vi "RITA_GUI.vi"() -> ()   [LabVIEW 2012]
uses:
  <vilib>/silver_ctls/ArrayMatrixCluster/Real Matrix NI_Silver.ctl
  State.ctl
  Signal Analysis.lvlib
  Report.lvlib
  Logger VIs.lvlib
  Pressure Regulator Controller.lvlib
  MultiClamp 700B Controls.lvlib
  Sciscan Scope Daemon.lvlib
  Autopatcher Daemon.lvlib
  Visual Analyser.lvlib
  Scientifica Manipulator Daemon.lvlib
  Targeting Unit.lvlib
  Signal Acquisition.lvlib
panel:
  in  "Start Coordinates [pix] 2":cluster{"X":dbl, "Y":dbl}
  out "Traced Objects [pix]":T1(array[cluster])
  out "All Objects [pix]":T1(array[cluster])
  in  "Traced Objects":i32
  in  "Start Coordinates [pix]":cluster{"X":dbl, "Y":dbl}
  in  "State":T2=enum."LOAD"
  in  "Autotune Gain":bool
  in  "Target Amplitude [V]":dbl
  in  "Main Tab Control":enum32{"Main", "Report", "Configuration"}(tab)
  in  "Target\nDistance [um]":dbl
  in  "Axial Approach":bool
  in  "Image construction":T3={"Delay"=1.0, "Display-N"=0, "Average"=0, "Frames"=10, "Zoom"=1.0, "Time\nStamp"=timestamp(0 s since 1904-01-01), "Auto Delay"=FALSE} {"Zoom" items=["1X"=1.0, "2X"=2.0, "3X"=3.0, "4X"=4.0, "5X"=5.0, "6X"=6.0, "7X"=7.0, "8X"=8.0]; "Average" items=["No Average", "Group Average", "Moving Average"]; "Delay" min=1.0 max=320.0 step=1.0 scale=1.0..320.0}
  out "Resistance [MOhm]":dbl format="%#_5g"
  out "Current [nA]":dbl format="%#_3g"
  in  "Gain":u16(ring)=1 items=["1"=1, "2"=2, "5"=5, "10"=10, "20"=20, "50"=50, "100"=100, "200"=200, "500"=500, "1000"=1000, "2000"=2000]
  in  "Manipulator":T4={"Indicator 7"={"Approach Indicator"=TRUE}, "Zero"=FALSE, "Step"=FALSE, "Drive to"=FALSE, "Current Position"={"X [um]"=0.0, "Y [um]"=0.0, "Z [um]"=0.0}, "Indicator 15"={"Status"=FALSE}, "Depth [um]"=0.0, "Destination Position"={"X [um]"=0.0, "Y [um]"=0.0, "Z [um]"=0.0}, "Go to"=FALSE, "Axial Approach"=TRUE, "Direction"=enum."Axial"}
  in  "Test Signal Parameters and Offset":T5 {"Frequency\n[hz]" items=["2 hz "=2, "5 hz"=5, "10 hz "=10, "20 hz"=20, "50 hz"=50, "60 hz"=60, "100 hz"=100, "200 hz"=200, "500 hz"=500, "1000 hz"=1000]}
  out "Test Signal":waveform(dbl)(graph)
  out "Resistance":T6(graph)
  out "Current":dbl(graph)
  in  "Pressure Controls":T7 {"Pressure Sp Manual [KPa]" scale=-50.0..100.0}
  in  "Holding Potential":T8 {"Holding Potential [mV]" scale=-100.0..100.0}
  in  "Signal Filter and PSD":T9
  in  "Dialog":cluster{"Indicator":bool}
  in  "High Level Controls":T10={"Record Button"=FALSE, "Exit"=FALSE, "Hunt"=FALSE, "Break In"=FALSE, "Seal"=FALSE, "Drive In"=FALSE, "Load Pipette"=FALSE, "REC"=FALSE, "File Path Control"=path "D:/Rita Logfiles", "Auto Button"=FALSE, "Auto"=FALSE, "Engage Target"=FALSE, "Abort"=FALSE}
  in  "Tip Acquisition":T11={"Focus Tip"=FALSE, "Acquire Tip"=FALSE, "Indicator 7"={"Tip Indicator"=FALSE}, "Tip Coordinates"={"X [um]"=nan, "Y [um]"=nan, "Z [um]"=nan}, "Disengage Tip"=FALSE}
  in  "Target Acquisition":T12={"Indicator 7"={"Target Indicator"=FALSE}, "Focus Target"=FALSE, "Acquire Target"=FALSE, "Target Coordinates"={"X [um]"=nan, "Y [um]"=nan, "Z [um]"=nan}, "Disengage Target"=FALSE}
  in  "Capacitance Compensation":T13
  out "Image":T14(plugin-control)
  in  "Resistance Levels":T15={"R0"=0.0, "R0/R1"=0.0, "R1"=0.0, "R1/R2"=0.0, "R2"=0.0, "R0-R2"=0.0, "R0/R2"=0.0, "Detect [%]"=10.0, "Break in "=100.0} {"Break in" scale=1.0..1000.0; "Detect [%]" scale=1.0..1000.0; "R0/R2" format="%.0f%%"; "R0-R2" scale=-100.0..100.0; "R2" scale=1.0..1000.0; "R1/R2" format="%.0f%%"; "R1" scale=1.0..1000.0; "R0/R1" format="%.0f%%"; "R0" scale=1.0..1000.0}
  in  "Scope Position":T16
  in  "Pipette Crash Indicator":cluster{"Pipette Crash":bool}
  in  "Align Trajectory":bool
  in  "Find Shank":bool
  in  "Find Tip":bool
  in  "Visualization Channels":T17={"Red\nChannel"={-29500.0, 275.0}, "Auto Adjust Red"=TRUE, "Green\nChannel"={-31433.0, -13386.0}, "Auto Adjust Green"=TRUE, "Visualized Color Plane"=8} {"Visualized Color Plane" items=["Red", "Green", "Blue", "Hue", "Saturation", "Luminance", "Value", "Intensity", "RGB"]; "Green\nChannel" scale=-32768.0..32767.0; "Red\nChannel" scale=-32768.0..32767.0}
  in  "Focus Button":bool
  in  "FOV":T18
  in  "Tab Control 2":enum32{"Analysis", "Calibration"}(tab)
  in  "Analisys and Tracking":T19={"Image Analisys"=TRUE, "Analysis\nPlane"=0, "Erosion\nFilter"=4, "Target Update Method"=0, "Objects"=0, "Target Update"=FALSE, "Object Tracking"=FALSE, "Traced\nObject\n[um]"={"X"=nan, "Y"=nan, "Z"=nan}, "Status"=FALSE, "Area"=0.0, "Cntr"=0.0} {"Target Update Method" items=["On Demand", "Continuos"]; "Erosion\nFilter" max=10 step=1 scale=0.0..10.0; "Analysis\nPlane" items=["Red", "Green", "Blue", "Hue", "Saturation", "Luminance", "Value", "Intensity"]}
  in  "Calibration Angles":T20={"Angles"={"Azimut"=-0.02262988105691686, "Elevation"=0.523611383535619}, "Calibrate Azimut"=FALSE, "Calibrate Elevation"=FALSE, "Autocalibration"=FALSE, "Acquire Initial Point"=FALSE, "Acquire Final Point"=FALSE} {"Angles"."Elevation" format="%#_10g"; "Angles"."Azimut" format="%#_10g"}
  in  "FOV Calibration":T21
  in  "Analyzer":bool=TRUE
  in  "Axial distance to cover [um]":dbl
  out "Logo":cluster{"Logo":picture}
  in  "Report Indicator":T22={"Report Plot"=FALSE, "File Path Control"=path "", "Resistance"=[], "Current"=[], "Current 2"=[], "Current 3"=[], "Position"=[], "Slider"=0.0, "Trajectory"=[], "Report Image"=refnum, "Play Button"=FALSE, "Report Visualization Options"={"Red\nChannel"={0.0, 7.070707070707071}, "Auto Adjust Red"=FALSE, "Green\nChannel"={0.0, 7.070707070707071}, "Auto Adjust Green"=FALSE, "Visualized Color Plane"=8, "Vision Overlay"=TRUE}, "Loading Bar"=0.0} {"Loading Bar" min=0.0 max=1.0 step=0.001 scale=0.0..1.0; "Report Visualization Options"."Visualized Color Plane" items=["Red", "Green", "Blue", "Hue", "Saturation", "Luminance", "Value", "Intensity", "RGB"]; "Report Visualization Options"."Green\nChannel" scale=-32768.0..32767.0; "Report Visualization Options"."Red\nChannel" scale=-32768.0..32767.0; "Slider" min=0.0 step=0.05 scale=0.0..600.0}
  in  "Geometrical Transformation Parameters":T24={"Scope Transformation Matrix"=[[1.0, 0.0], [0.0, 1.0]], "Manipulator transformation"=[[-1.0], [-1.0], [-1.0]], "Coorection Factor"={"Kx"=1.0, "Ky"=1.0, "Kz"=1.0}} {"Coorection Factor"."Kz" format="%#_10g"; "Coorection Factor"."Ky" format="%#_10g"; "Coorection Factor"."Kx" format="%#_10g"}
  in  "Calibration Parameters":T25={"Test Signal"={"Break In"={"Amplitude [mV]"=30, "Frequency [hz]"=100}, "Extracellular"={"Amplitude [mV]"=10, "Frequency [hz]"=100}}, "Capacitance Compensation"={"Iterations"=2, "Timeout [ms]"=3000}, "Holding Potential Dynamics"={"Start [mV]"=-70.0, "Target [mV]"=-70.0, "Speed [mV/s]"=2.0}, "Manipulator Dynamics"={"Step length [um]"=2.0, "Interstep Interval [ms]"=1500, "Initial Speed [um/s]"=10.0, "Max Speed [um/s]"=10.0, "Acceleration [um/s^2]"=10.0, "Max Depth [um]"=1200.0, "Max Penetration [um]"=1200.0}, "Suction Parameters"={"Initial Pressure [Kpa]"=-5.0, "Minimum Pressure [KPa]"=-25.0, "Decremental Step [KPa]"=-5.0, "Decremental Threshold [%]"=5.0, "Falloff Threshold [%]"=50.0, "Falloff Lag [ms]"=3000.0, "Monitor Refresh [ms]"=1000.0}, "Pressure SPs [KPa]"={"High"=50.0, "Low"=10.0}, "Seal Parameters"={"Seal Target [MOhm]"=1000.0, "Stability Threhsold [%]"=10.0, "Seal Timeout [s]"=600.0, "Stability Refresh [ms]"=1000.0}, "Break in pulse Dynamics"={"Length [ms]"=250.0, "Voltage [mV]"=1000.0, "Pressure [KPa]"=-25.0}, "Unblockage Parameters"={"Blockage Threshold [%]"=10.0, "Max Attempt"=3}, "Targeter Settings"={"Approaching Calibration"={"Approach Factor [um]"=0.9, "Final Clearance [um]"=2.0}, "Optic Flow Settings"={"Pyramid Levels"=6, "Max Iterations"=8, "Displacement Threshold"=0.0, "Window Size"=45}, "Focus"={"Timeout [ms]"=5000, "Max Attempts"=2, "Method"=enum."Continuous"}}} {"Test Signal"."Extracellular"."Frequency [hz]" items=["2 hz "=2, "5 hz"=5, "10 hz "=10, "20 hz"=20, "50 hz"=50, "60 hz"=60, "100 hz"=100, "200 hz"=200, "500 hz"=500, "1000 hz"=1000]; "Test Signal"."Break In"."Frequency [hz]" items=["2 hz "=2, "5 hz"=5, "10 hz "=10, "20 hz"=20, "50 hz"=50, "60 hz"=60, "100 hz"=100, "200 hz"=200, "500 hz"=500, "1000 hz"=1000]}
  in  "Hardware Configuration":T26={"Pressure Controller Dynamics"={"Positive Branch"={"Kp"=0.05, "Ki"=1.0, "Kd"=1e-06}, "Negative Branch"={"Kp"=1.0, "Ki"=10.0, "Kd"=1e-06}}, "Amplifier"={"Multiclamp Serial Number"="00832548", "Multiclamp Channel"=0}, "Manipulator Port"="COM10", "Objective"=600, "Sciscan core Ref"=path "C:/Users/Southampton/Desktop/LUCA_SciScan_141211/GFG/GFG_core.ref", "Signals Sampling"={"Sample Mode"=10123, "Sampling frequecy [hz]"=20000.0, "Samples Number"=1000}, "Electrode Signals"={"Scale Type"=10348, "Terminal Configuration"=10083, "Scale Name"="", "Range [V]"={"max"=10.0, "min"=-10.0}, "Channel 2 [Potential]"="Dev4/ai1", "Channel 1 [Current]"="Dev4/ai2"}, "Pressure Signal"={"Scale Type"=10065, "Terminal Configuration"=10083, "Scale Name"="Compund Pressure", "Range [V]"={"max"=4.0, "min"=0.0}, "Physical Channel"="Dev4/ai4"}, "IIR Filter Specifications"={"Topology"=enum."Off", "Type"=enum."Lowpass", "Order"=0, "Lower Fc"=0.0, "Upper Fc"=0.0, "PB Ripple"=0.0, "SB Attenuation"=0.0}, "Pressure Controller Port"="COM8", "Scope Dynamics"={"Initial Speed [um/s]"=500.0, "Max Speed [um/s]"=1000.0, "Acceleration [um/s^2]"=25.0, "Max Depth [um]"=5000.0}} {"Pressure Signal"."Terminal Configuration" items=["Default"=-1, "RSE"=10083, "Differential"=10106, "Pseudodifferential"=12529]; "Pressure Signal"."Scale Type" items=["Volts"=10348, "Custom Scale"=10065]; "Electrode Signals"."Terminal Configuration" items=["Default"=-1, "RSE"=10083, "Differential"=10106, "Pseudodifferential"=12529]; "Electrode Signals"."Scale Type" items=["Volts"=10348, "Custom Scale"=10065]; "Signals Sampling"."Sample Mode" items=["Finite Samples"=10178, "Continuous Samples"=10123, "Hardware Timed Single Point"=12522]; "Objective" items=["Nikon 16x / 0.80w"=600]; "Amplifier"."Multiclamp Channel" items=["Channel 1", "Channel 2"]}
  in  "Pipette Search":T27={"Stability Delay [ms]"=1000, "Scan Area"={"Lateral [um]"=1200.0, "Vertical [um]"=1600.0}, "Vertical Sections"=10, "Scanning Direction"={"X"=0, "Y"=1, "Z"=1}, "Fucusing step [um]"=-30.0, "Erosion Value"=3} {"Scanning Direction"."Z" items=["Negative"=-1, "Positive"=1]; "Scanning Direction"."Y" items=["Negative"=-1, "Fixed"=0, "Positive"=1]; "Scanning Direction"."X" items=["Negative"=-1, "Fixed"=0, "Positive"=1]}
  in  "Configuration Files":T28
  out "Error Out":errorcluster
  # "Image"
  # "Test signal and offset"
  # "Capacitance Compensation"
  # "Visualization"
  # "Analysis and Tracking"
  # "Calibration Angles"
  # "Visualization"
  # "Xv"
  # "Yv"
  # "Xscope"
  # "Yscope"
  # "axial direction (exiting -1 entering +1)"
  # "Flip System of Reference (Yes -1 No 1)"
  # "Insertion step Sign"
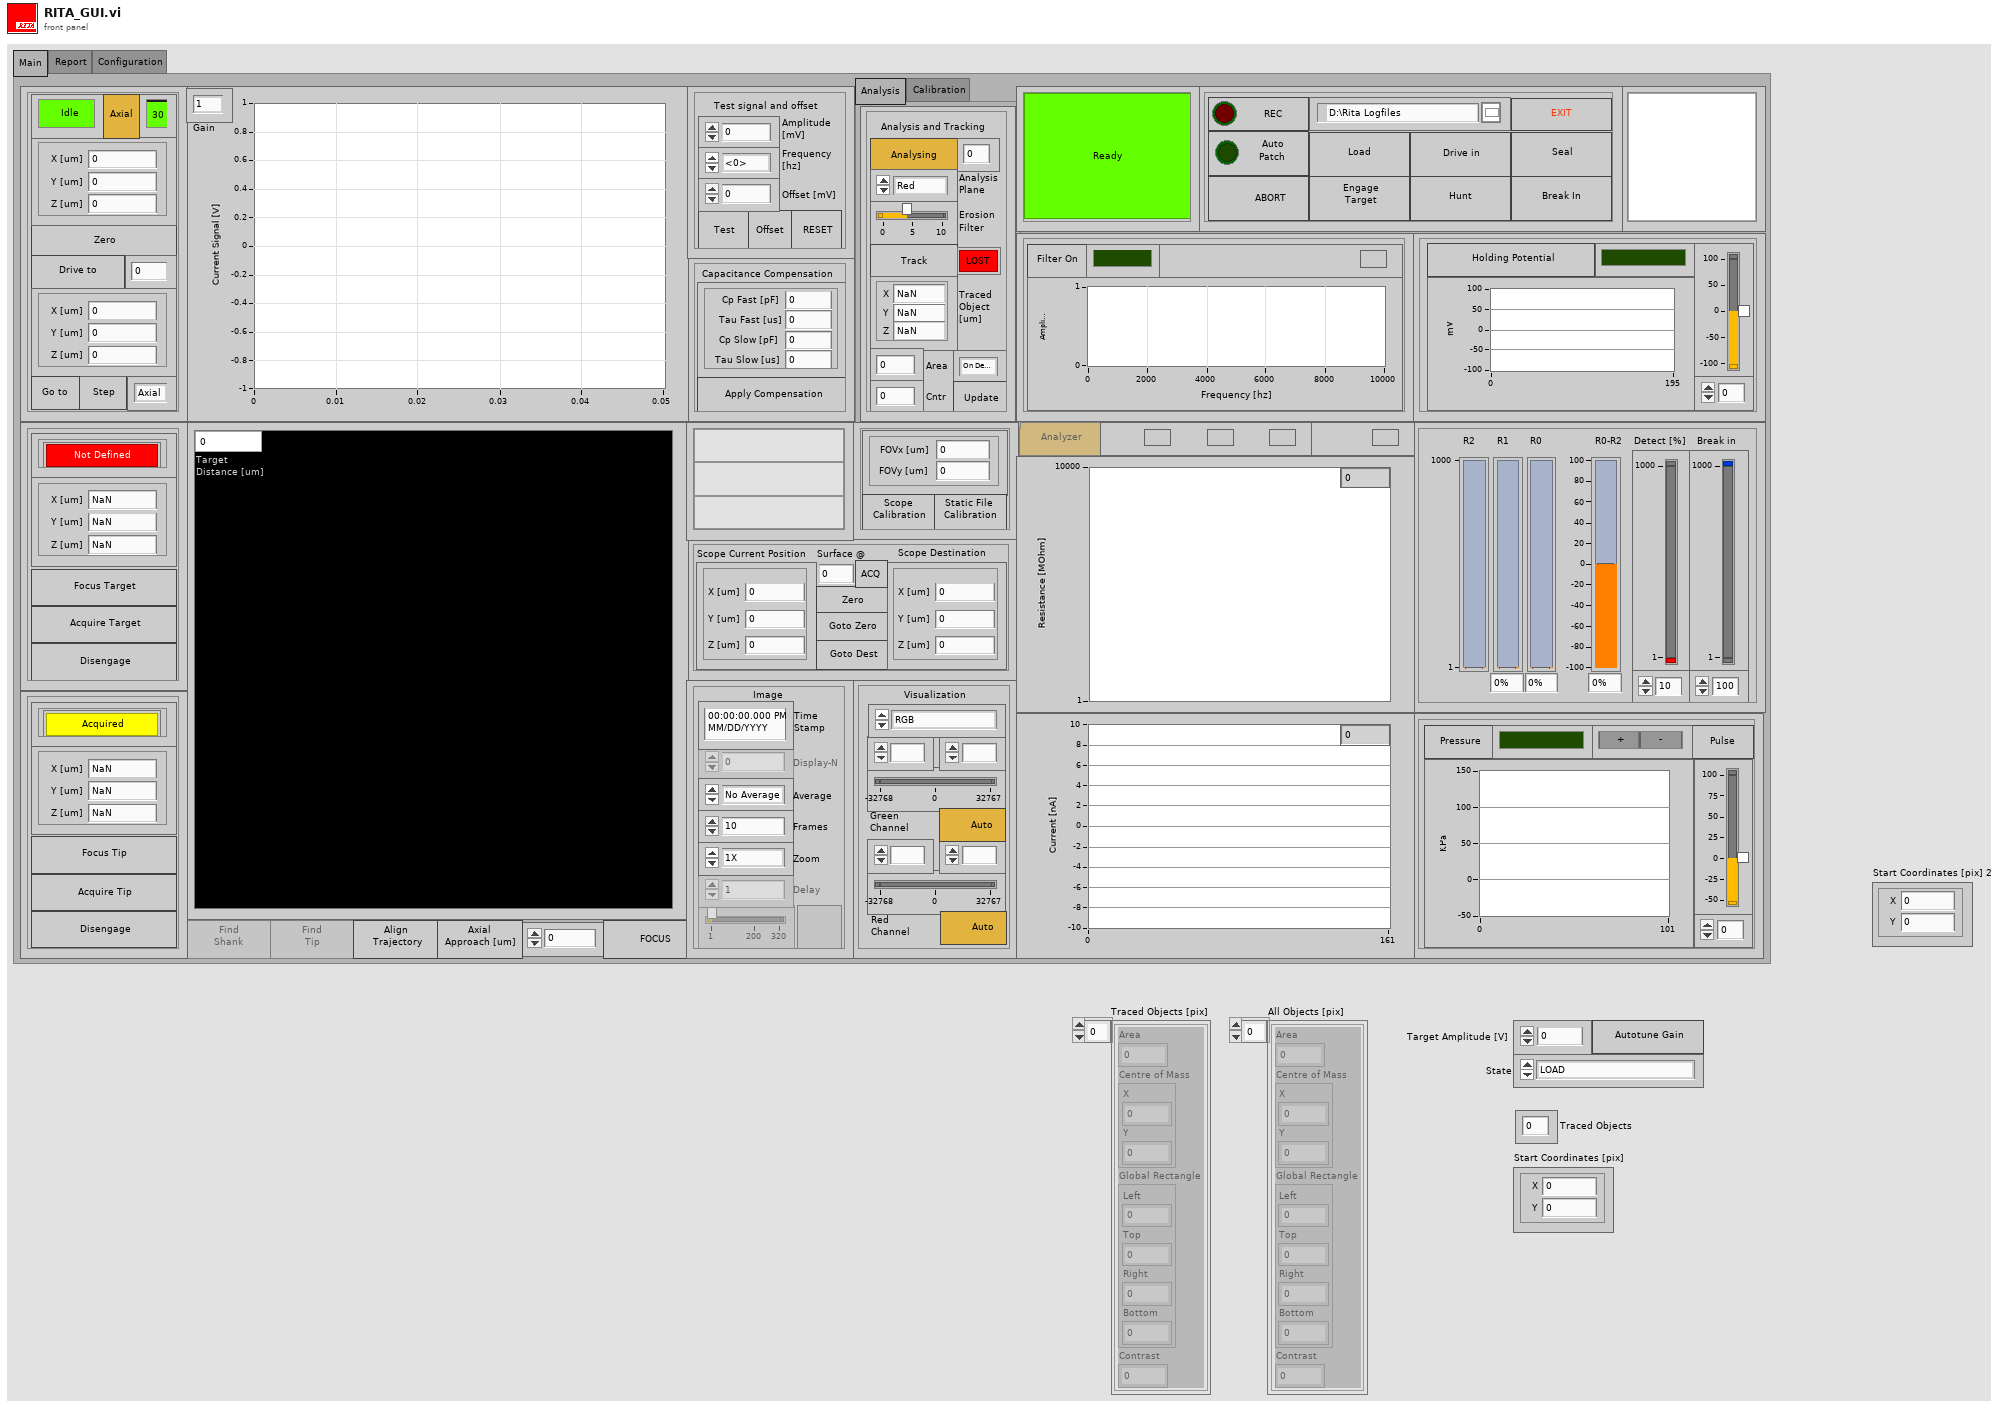
[diagram p1: front panel]
types:
  T1 = cluster{"Area":dbl, "Centre of Mass":cluster{"X":dbl, "Y":dbl}, "Global Rectangle":cluster{"Left":dbl, "Top":dbl, "Right":dbl, "Bottom":dbl}, "Contrast":dbl}[]
  T2 = typedef "State.ctl" = enum16{"READY", "LOAD", "LOCALIZATION", "HUNTING", "SEAL", "BREAKIN", "WCR", "ALIGN", "APPROACH", "TARGETING"}
  T3 = cluster{"Delay":dbl, "Display-N":i8, "Average":u16, "Frames":i8, "Zoom":dbl, "Time\nStamp":timestamp, "Auto Delay":bool}
  T4 = cluster{"Indicator 7":cluster{"Approach Indicator":bool}, "Zero":bool, "Step":bool, "Drive to":bool, "Current Position":cluster{"X [um]":dbl, "Y [um]":dbl, "Z [um]":dbl}, "Indicator 15":cluster{"Status":bool}, "Depth [um]":dbl, "Destination Position":cluster{"X [um]":dbl, "Y [um]":dbl, "Z [um]":dbl}, "Go to":bool, "Axial Approach":bool, "Direction":enum16{"Z", "Axial"}}
  T5 = cluster{"Pipette Offset":bool, "Test Signal":bool, "Amplitude\n[mV]":i32, "Frequency\n[hz]":u16, "Offset [mV]":dbl, "Reset":bool}
  T6 = cluster{"Value":dbl, "Value 2":dbl, "Value 3":dbl}
  T7 = cluster{"Activate Pressure":bool, "Pulse":bool, "Indicator 16":cluster{"Valves":bool}, "Indicator 17":cluster{"Positive Branch":bool, "Negative Branch":bool}, "Pressure Sp Manual [KPa]":dbl, "Pressure Signal":dbl}
  T8 = cluster{"Holding Potential Chart":dbl, "Holding Potential":bool, "HP Indicator":cluster{"Holding Potential Led":bool}, "Holding Potential [mV]":i32}
  T9 = cluster{"Filter":bool, "Indicator 18":cluster{"Filter Led Indicator":bool}, "PSD 2":cluster{"f0":dbl, "df":dbl, "magnitude":dbl[]}}
  T10 = cluster{"Record Button":bool, "Exit":bool, "Hunt":bool, "Break In":bool, "Seal":bool, "Drive In":bool, "Load Pipette":bool, "REC":bool, "File Path Control":path, "Auto Button":bool, "Auto":bool, "Engage Target":bool, "Abort":bool}
  T11 = cluster{"Focus Tip":bool, "Acquire Tip":bool, "Indicator 7":cluster{"Tip Indicator":bool}, "Tip Coordinates":cluster{"X [um]":dbl, "Y [um]":dbl, "Z [um]":dbl}, "Disengage Tip":bool}
  T12 = cluster{"Indicator 7":cluster{"Target Indicator":bool}, "Focus Target":bool, "Acquire Target":bool, "Target Coordinates":cluster{"X [um]":dbl, "Y [um]":dbl, "Z [um]":dbl}, "Disengage Target":bool}
  T13 = cluster{"Capacitance Compensation Indicators":cluster{"Cp Fast [pF]":dbl, "Tau Fast [us]":dbl, "Cp Slow [pF]":dbl, "Tau Slow [us]":dbl}, "Capacitance Compensation":bool}
  T14 = typedef "IMAQ Image.ctl" = refnum<image>
  T15 = cluster{"R0":dbl, "R0/R1":dbl, "R1":dbl, "R1/R2":dbl, "R2":dbl, "R0-R2":dbl, "R0/R2":dbl, "Detect [%]":dbl, "Break in ":dbl}
  T16 = cluster{"Scope Current Position":cluster{"X [um]":dbl, "Y [um]":dbl, "Z [um]":dbl}, "Scope Zero":bool, "Drive to Zero":bool, "Drive to Position":bool, "Scope Destination":cluster{"X [um]":dbl, "Y [um]":dbl, "Z [um]":dbl}, "Surface @":dbl, "Acquire Surface":bool}
  T17 = cluster{"Red\nChannel":cluster{dbl, dbl}, "Auto Adjust Red":bool, "Green\nChannel":cluster{dbl, dbl}, "Auto Adjust Green":bool, "Visualized Color Plane":i32}
  T18 = cluster{"FOV indicator":cluster{"FOVx [um]":dbl, "FOVy [um]":dbl}, "Internal Calibration":bool, "Load Calibration File":bool}
  T19 = cluster{"Image Analisys":bool, "Analysis\nPlane":i32, "Erosion\nFilter":u32, "Target Update Method":i32, "Objects":i32, "Target Update":bool, "Object Tracking":bool, "Traced\nObject\n[um]":cluster{"X":dbl, "Y":dbl, "Z":dbl}, "Status":bool, "Area":dbl, "Cntr":dbl}
  T20 = cluster{"Angles":cluster{"Azimut":dbl, "Elevation":dbl}, "Calibrate Azimut":bool, "Calibrate Elevation":bool, "Autocalibration":bool, "Acquire Initial Point":bool, "Acquire Final Point":bool}
  T21 = cluster{"Calibrate FOV":bool, "Save current FOV":bool}
  T22 = cluster{"Report Plot":bool, "File Path Control":path, "Resistance":dynamicdata, "Current":dynamicdata, "Current 2":dynamicdata, "Current 3":dynamicdata, "Position":dynamicdata, "Slider":dbl, "Trajectory":cluster{"Y":dbl[], "Y":dbl[]}[], "Report Image":T14, "Play Button":bool, "Report Visualization Options":cluster{"Red\nChannel":cluster{dbl, dbl}, "Auto Adjust Red":bool, "Green\nChannel":cluster{dbl, dbl}, "Auto Adjust Green":bool, "Visualized Color Plane":i32, "Vision Overlay":bool}, "Loading Bar":dbl}
  T23 = typedef "Real Matrix NI_Silver.ctl" = dbl[][]
  T24 = cluster{"Scope Transformation Matrix":T23, "Manipulator transformation":T23, "Coorection Factor":cluster{"Kx":dbl, "Ky":dbl, "Kz":dbl}}
  T25 = cluster{"Test Signal":cluster{"Break In":cluster{"Amplitude [mV]":i32, "Frequency [hz]":u16}, "Extracellular":cluster{"Amplitude [mV]":i32, "Frequency [hz]":u16}}, "Capacitance Compensation":cluster{"Iterations":i32, "Timeout [ms]":u32}, "Holding Potential Dynamics":cluster{"Start [mV]":dbl, "Target [mV]":dbl, "Speed [mV/s]":dbl}, "Manipulator Dynamics":cluster{"Step length [um]":dbl, "Interstep Interval [ms]":u32, "Initial Speed [um/s]":dbl, "Max Speed [um/s]":dbl, "Acceleration [um/s^2]":dbl, "Max Depth [um]":dbl, "Max Penetration [um]":dbl}, "Suction Parameters":cluster{"Initial Pressure [Kpa]":dbl, "Minimum Pressure [KPa]":dbl, "Decremental Step [KPa]":dbl, "Decremental Threshold [%]":dbl, "Falloff Threshold [%]":dbl, "Falloff Lag [ms]":dbl, "Monitor Refresh [ms]":dbl}, "Pressure SPs [KPa]":cluster{"High":dbl, "Low":dbl}, "Seal Parameters":cluster{"Seal Target [MOhm]":dbl, "Stability Threhsold [%]":dbl, "Seal Timeout [s]":dbl, "Stability Refresh [ms]":dbl}, "Break in pulse Dynamics":cluster{"Length [ms]":dbl, "Voltage [mV]":dbl, "Pressure [KPa]":dbl}, "Unblockage Parameters":cluster{"Blockage Threshold [%]":dbl, "Max Attempt":i32}, "Targeter Settings":cluster{"Approaching Calibration":cluster{"Approach Factor [um]":dbl, "Final Clearance [um]":dbl}, "Optic Flow Settings":cluster{"Pyramid Levels":i32, "Max Iterations":i32, "Displacement Threshold":dbl, "Window Size":i32}, "Focus":cluster{"Timeout [ms]":u32, "Max Attempts":u32, "Method":enum16{"Continuous", "On Demand"}}}}
  T26 = cluster{"Pressure Controller Dynamics":cluster{"Positive Branch":cluster{"Kp":dbl, "Ki":dbl, "Kd":dbl}, "Negative Branch":cluster{"Kp":dbl, "Ki":dbl, "Kd":dbl}}, "Amplifier":cluster{"Multiclamp Serial Number":string, "Multiclamp Channel":u16}, "Manipulator Port":refnum<visa-resource-name>, "Objective":i16, "Sciscan core Ref":path, "Signals Sampling":cluster{"Sample Mode":i32, "Sampling frequecy [hz]":dbl, "Samples Number":i32}, "Electrode Signals":cluster{"Scale Type":i32, "Terminal Configuration":i32, "Scale Name":tag, "Range [V]":cluster{"max":dbl, "min":dbl}, "Channel 2 [Potential]":tag, "Channel 1 [Current]":tag}, "Pressure Signal":cluster{"Scale Type":i32, "Terminal Configuration":i32, "Scale Name":tag, "Range [V]":cluster{"max":dbl, "min":dbl}, "Physical Channel":tag}, "IIR Filter Specifications":cluster{"Topology":enum16{"Off", "Butterworth", "Chebyshev", "Inverse Chebyshev", "Elliptic", "Bessel"}, "Type":enum16{"Lowpass", "Highpass", "Bandpass", "Bandstop"}, "Order":i32, "Lower Fc":dbl, "Upper Fc":dbl, "PB Ripple":dbl, "SB Attenuation":dbl}, "Pressure Controller Port":refnum<visa-resource-name>, "Scope Dynamics":cluster{"Initial Speed [um/s]":dbl, "Max Speed [um/s]":dbl, "Acceleration [um/s^2]":dbl, "Max Depth [um]":dbl}}
  T27 = cluster{"Stability Delay [ms]":u32, "Scan Area":cluster{"Lateral [um]":dbl, "Vertical [um]":dbl}, "Vertical Sections":u32, "Scanning Direction":cluster{"X":i16, "Y":i16, "Z":i16}, "Fucusing step [um]":dbl, "Erosion Value":u32}
  T28 = cluster{"File Path Control":path, "Save current Configuration":bool, "Save current Configuration 2":bool}
  T29 = cluster{"Indicators":cluster{"Current Pos":refnum<vi>, "Destination":refnum<vi>, "Status":refnum<vi>, "Axial Approach":refnum<vi>}, "Settings":cluster{"Dynamics":refnum<vi>, "Transformation":refnum<vi>, "Direction":refnum<vi>}, "Controls":cluster{"Zero":refnum<vi>, "Step":refnum<vi>, "Drive To":refnum<vi>, "Go To":refnum<vi>, "Axial":refnum<vi>, "Depth [um]":refnum<vi>}}
  T30 = cluster{"Load Pipette":refnum<vi>, "Drive In":refnum<vi>, "Hunt":refnum<vi>, "Seal":refnum<vi>, "Break In":refnum<vi>, "Abort":refnum<vi>, "Exit":refnum<vi>, "Auto":refnum<vi>, "Auto Button":refnum<vi>}
  T31 = cluster{"Status":refnum<vi>, "Position":refnum<vi>, "Zero":refnum<vi>, "Step":refnum<vi>, "Localize":refnum<vi>, "Approach Indicator":refnum<vi>, "Depth [um]":refnum<vi>, "Drive to Zero":refnum<vi>, "Direction":refnum<vi>}
  T32 = cluster{"Zero":refnum<vi>, "Step":refnum<vi>, "Go to":refnum<vi>, "Drive to Depth":refnum<vi>, "Exit":refnum<vi>, "Abort":refnum<vi>, "Depth [um]":refnum<vi>, "Dest Position":refnum<vi>, "Axial":refnum<vi>, "Direction":refnum<vi>}
  T33 = cluster{"Current":refnum<vi>, "Holding Potential":refnum<vi>, "Recording indicator":refnum<vi>, "Pressure":refnum<vi>, "Resistance":refnum<vi>, "Manipulator Position":refnum<vi>, "Tip Coordinates":refnum<vi>, "Target Coordinates":refnum<vi>, "Surface in Space [um]":refnum<vi>, "State":refnum<vi>}
  T34 = cluster{"Current Signal":refnum<vi>, "PSD":refnum<vi>, "Pressure Signal":refnum<vi>, "Current [nA]":refnum<vi>, "Resistance [MOhm]":refnum<vi>}
  T35 = cluster{"Current Pos":refnum<vi>, "Image interface":refnum<vi>, "Transformation Matrix":refnum<vi>, "Zero":refnum<vi>, "Destination":refnum<vi>, "Drive to Position":refnum<vi>, "Zoom":refnum<vi>}
  T36 = cluster{"Focused Plane":cluster{"Focus":refnum<vi>, "Timeout":refnum<vi>, "Max Attempts":refnum<vi>, "Method":refnum<vi>}, "Time Stamp":refnum<vi>, "Visual Target":cluster{"Coordinates [um]":refnum<vi>, "Status":refnum<vi>, "Update":refnum<vi>, "Update Method":refnum<vi>, "Start Coordinates [pix]":refnum<vi>, "Area":refnum<vi>, "Contrast":refnum<vi>}, "Visible Objects [pix]":refnum<vi>}
  T37 = cluster{"Object Tracking Command":refnum<vi>, "Status Indicator":refnum<vi>, "Start Coordinates [pix]":refnum<vi>, "Traced Object [um]":refnum<vi>, "Area":refnum<vi>, "Contrast":refnum<vi>}
  T38 = cluster{"On/Off":refnum<vi>, "All Objects":refnum<vi>, "Color Plane":refnum<vi>, "Erosion":refnum<vi>, "Traced Objects":refnum<vi>, "Frame Time Stamp":refnum<vi>, "Optic Flow Settings":refnum<vi>, "All Object [pix]":refnum<vi>, "Traced Object [pix]":refnum<vi>}
  T39 = cluster{"Exit":refnum<vi>, "Abort":refnum<vi>, "Align Trajectory":refnum<vi>, "Axial Approach":refnum<vi>, "Dialog Indicator":refnum<vi>, "Approach Target":refnum<vi>, "Target\nDistance [um]":refnum<vi>, "Axial distance\nto cover [um]":refnum<vi>}
  T40 = cluster{"Coordinates":refnum<vi>, "Acquire":refnum<vi>, "Disengage":refnum<vi>, "Indicator":refnum<vi>, "Focus Target":refnum<vi>}
  T41 = cluster{"Coordinates":refnum<vi>, "Acquire":refnum<vi>, "Disengage":refnum<vi>, "Indicator":refnum<vi>, "Focus Tip":refnum<vi>}
  T42 = cluster{"Pulse Dynamics":cluster{"Length [ms]":refnum<vi>, "Pressure [KPa] Closed Loop":refnum<vi>, "Voltage [mV] Open Loop":refnum<vi>}, "On/Off":refnum<vi>, "Exit":refnum<vi>, "Pulse":refnum<vi>, "Pressure Sp [KPa]":refnum<vi>, "Pressure Controller Dynamics":refnum<vi>}
  T43 = cluster{"Focus Tip":refnum<vi>, "Focus Target":refnum<vi>, "Drive to Zero":refnum<vi>, "Zero":refnum<vi>, "Acquire Tip":refnum<vi>, "Focus Button":refnum<vi>, "Exit":refnum<vi>, "Abort":refnum<vi>, "Drive to":refnum<vi>, "Surface @":refnum<vi>, "Acquire Surface":refnum<vi>}
  T44 = cluster{"Angles":refnum<vi>, "Calibration":refnum<vi>, "Transformation":refnum<vi>}
  T45 = cluster{"Display Every N":refnum<vi>, "Average":refnum<vi>, "Frames":refnum<vi>, "Colour Plane":refnum<vi>, "Zoom":refnum<vi>, "Delay":refnum<vi>, "Equalization":cluster{"Green Channel":refnum<vi>, "Auto Adjust Green":refnum<vi>, "Red Channel":refnum<vi>, "Auto Adjust Red":refnum<vi>}, "Auto Delay":refnum<vi>}
  T46 = cluster{"Resistance":refnum<vi>, "Current":refnum<vi>, "Pressure":refnum<vi>, "Holding Potential":refnum<vi>, "Position":refnum<vi>, "Trajectory":refnum<vi>}
  T47 = cluster{"Indicators":cluster{"FOV":refnum<vi>, "Angles":refnum<vi>}, "Buttons":cluster{"Cal FOV":refnum<vi>, "Cal Azimut":refnum<vi>, "Cal Elevation":refnum<vi>, "Auto Cal":refnum<vi>, "Acq Initial":refnum<vi>, "Acq Final":refnum<vi>}, "Stability Delay [ms]":refnum<vi>, "Scale Coorection Factor":refnum<vi>}
  T48 = cluster{"Valves":refnum<vi>, "Branch +":refnum<vi>, "Branch -":refnum<vi>}
  T49 = cluster{"Length [ms]":refnum<vi>, "Pressure [KPa] Closed Loop":refnum<vi>, "Voltage [mV] Open Loop":refnum<vi>}
  T50 = cluster{"Approach  Factor":refnum<vi>, "Final Clearance":refnum<vi>}
  T51 = cluster{"Approach":refnum<vi>, "Status":refnum<vi>, "Current Position":refnum<vi>}
  T52 = cluster{"Dynamics":refnum<vi>, "Transformation":refnum<vi>}
  T53 = cluster{"Tip Coordinates":refnum<vi>, "Target Coordinates":refnum<vi>, "Scope Position":refnum<vi>, "FOV":refnum<vi>, "Scope Goto Position":refnum<vi>}
  T54 = cluster{"Find Shank":refnum<vi>, "Find Tip":refnum<vi>, "Scanning Direction":refnum<vi>, "Scan Area":refnum<vi>, "Stability Delay [ms]":refnum<vi>, "Vertical Steps":refnum<vi>, "Fucusing step [um]":refnum<vi>, "Erosion Value":refnum<vi>}
  T55 = cluster{"Angles":refnum<vi>, "Objective Diameter":refnum<vi>, "Pipette Crash":refnum<vi>}
  T56 = cluster{"Internal Calibrated FOV":refnum<vi>, "Load FOV calibration file":refnum<vi>, "Save current FOV":refnum<vi>}
  T57 = cluster{"On/Off":refnum<vi>, "Filter On/Off":refnum<vi>, "Exit":refnum<vi>, "IIR filter specifications":refnum<vi>}
  T58 = cluster{"Suction Parameters":refnum<vi>, "Holding Potential Dynamics":refnum<vi>, "Seal Parameters":refnum<vi>}
  T59 = cluster{"Test Signal Levels":refnum<vi>, "Pressure Levels [KPa]":refnum<vi>}
  T60 = cluster{"ON/OFF":refnum<vi>, "Controller [mV]":refnum<vi>}
  T61 = cluster{"Autotune Gain":refnum<vi>, "Target Amplitude [V]":refnum<vi>}
  T62 = cluster{"R(Z=0)":refnum<vi>, "R(Z=-1)":refnum<vi>, "R(Z=-2)":refnum<vi>, "R0-R2":refnum<vi>, "R0/R2 [%]":refnum<vi>, "R1/R2 [%]":refnum<vi>, "R0/R1 [%]":refnum<vi>}
  T63 = cluster{"Pipette Offset":refnum<vi>, "Offset":refnum<vi>, "Test Signal":refnum<vi>, "Amplitude [mV]":refnum<vi>, "Frequency [hz]":refnum<vi>}
  T64 = cluster{"Blockage Threshold":refnum<vi>, "Max Attempt":refnum<vi>}
  T65 = cluster{"On/Off":refnum<vi>, "Resistance [MOhm]":refnum<vi>, "Current [pA]":refnum<vi>}
  T66 = cluster{"On/Off":refnum<vi>, "Pulse Controls":cluster{"Pulse":refnum<vi>, "Length [ms]":refnum<vi>, "Voltage [mV]":refnum<vi>, "Pulse Pressure [KPa]":refnum<vi>}, "Pressure Sp Manual [KPa]":refnum<vi>}
  T67 = cluster{"Holding Potential [mV]":refnum<vi>, "Holding Potential":refnum<vi>, "Holding Potential Indicator":refnum<vi>, "Holding Potential Led":refnum<vi>}
  T68 = cluster{"Timeout [ms]":refnum<vi>, "Iterations":refnum<vi>, "Compensate":refnum<vi>, "Capacitance Compensation Indicators":refnum<vi>}
  T69 = cluster{"Autotune Gain":refnum<vi>, "Target Amplitude [mV]":refnum<vi>}
  T70 = cluster{"Test Signal":refnum<vi>, "Amplitude [mV]":refnum<vi>, "Frequency [hz]":refnum<vi>}
  T71 = cluster{"Pipette Offset":refnum<vi>, "Offset Value [mV]":refnum<vi>}
  T72 = cluster{"Sample Mode":i32, "Sampling frequecy [hz]":dbl, "Samples Number":i32}
  T73 = cluster{"Scale Type":i32, "Terminal Configuration":i32, "Scale Name":tag, "Range [V]":cluster{"max":dbl, "min":dbl}, "Physical Channel":tag}
  T74 = cluster{"Scale Type":i32, "Terminal Configuration":i32, "Scale Name":tag, "Range [V]":cluster{"max":dbl, "min":dbl}, "Channel 2 [Potential]":tag, "Channel 1 [Current]":tag}
  T75 = cluster{"Object Tracking Command":refnum<vi>, "Status Indicator":refnum<vi>, "Start Coordinates [pix]":refnum<vi>, "Traced Object [um]":refnum<vi>, "Area":refnum<vi>, "Contrast":refnum<vi>}[]
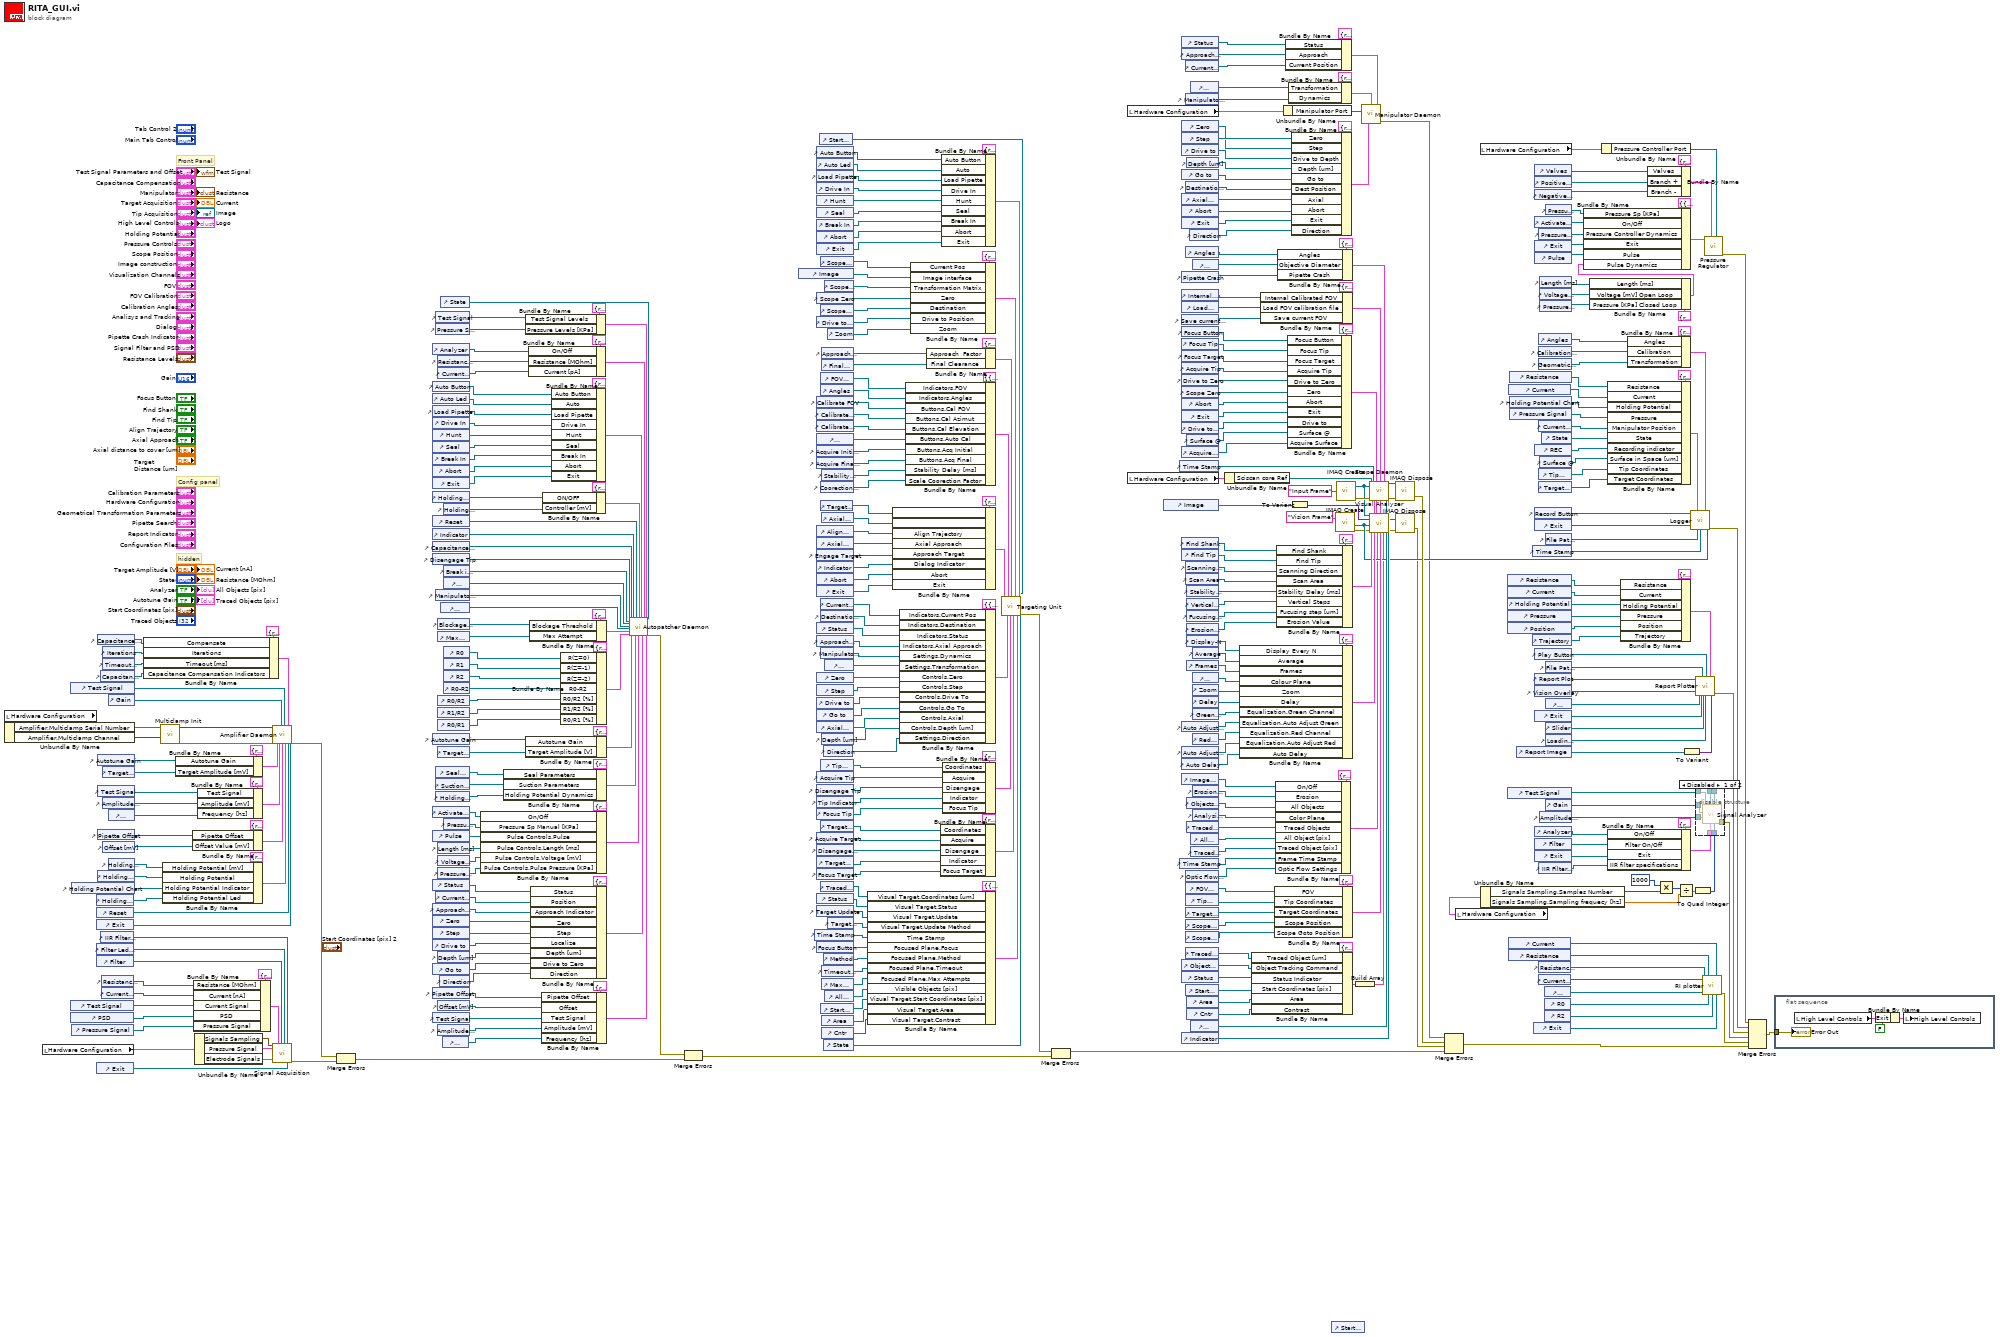
[diagram p0: block diagram]
diagram:
  # "hidden"
  # "Config panel"
  # "Front Panel"
  n1 = local read "Hardware Configuration"() -> (w408:T26)
  n2 = Unbundle By Name(w408) -> ("Amplifier.Multiclamp Serial Number"=w407:string, "Amplifier.Multiclamp Channel"=w401:u16)
  n3 = local read "Hardware Configuration"() -> (w88:T26)
  n4 = control-ref of="Test Signal"() -> (w93:refnum<vi>)
  n5 = control-ref of="PSD"() -> (w46:refnum<vi>)
  n6 = control-ref of="Test Signal"() -> (w411:refnum<vi>)
  n7 = control-ref of="Pressure Signal"() -> (w92:refnum<vi>)
  n8 = control-ref of="Holding Potential Chart"() -> (w420:refnum<vi>)
  n9 = control-ref of="Holding Potential Led"() -> (w402:refnum<vi>)
  n10 = control-ref of="Reset"() -> (w400:refnum<vi>)
  n11 = control-ref of="Exit"() -> (w423:refnum<vi>)
  n12 = control-ref of="Filter Led Indicator"() -> (w95:refnum<vi>)
  n13 = control-ref of="Filter"() -> (w94:refnum<vi>)
  n14 = control-ref of="Exit"() -> (w97:refnum<vi>)
  n15 = control-ref of="Capacitance Compensation"() -> (w419:refnum<vi>)
  n16 = control-ref of="Autotune Gain"() -> (w405:refnum<vi>)
  n17 = control-ref of="Test Signal"() -> (w413:refnum<vi>)
  n18 = control-ref of="Pipette Offset"() -> (w416:refnum<vi>)
  n19 = control-ref of="Holding Potential"() -> (w421:refnum<vi>)
  n20 = control-ref of="IIR Filter Specifications"() -> (w96:refnum<vi>)
  n21 = control-ref of="Capacitance Compensation Indicators"() -> (w410:refnum<vi>)
  n22 = control-ref of="Resistance [MOhm]"() -> (w41:refnum<vi>)
  n23 = control-ref of="Current [nA]"() -> (w42:refnum<vi>)
  n24 = control-ref of="Iterations"() -> (w418:refnum<vi>)
  n25 = control-ref of="Timeout [ms]"() -> (w409:refnum<vi>)
  n26 = control-ref of="Target Amplitude [V]"() -> (w406:refnum<vi>)
  n27 = control-ref of="Amplitude [mV]"() -> (w415:refnum<vi>)
  n28 = control-ref of="Offset [mV]"() -> (w417:refnum<vi>)
  n29 = control-ref of="Gain"() -> (w412:refnum<vi>)
  n30 = control-ref of="Frequency [hz]"() -> (w414:refnum<vi>)
  n31 = control-ref of="Holding Potential [mV]"() -> (w422:refnum<vi>)
  n32 = Bundle By Name(cluster=T68 {"Timeout [ms]"=refnum, "Iterations"=refnum, "Compensate"=refnum, "Capacitance Compensation Indicators"=refnum} ("Capacitance Compensation"), "Compensate"=w419, "Iterations"=w418, "Timeout [ms]"=w409, "Capacitance Compensation Indicators"=w410) -> (w431:T68)
  n33 = call "Multiclamp Init.vi"("Channel"=w401, "pszSerialNum"=w407) -> ("error out"=w90:errorcluster, "Handler"=w89:i32)  [unwired: 7 in, 1 out]
  n34 = Bundle By Name(cluster=T67 {"Holding Potential [mV]"=refnum, "Holding Potential"=refnum, "Holding Potential Indicator"=refnum, "Holding Potential Led"=refnum} ("Holding Potential"), "Holding Potential [mV]"=w422, "Holding Potential"=w421, "Holding Potential Indicator"=w420, "Holding Potential Led"=w402) -> (w403:T67)
  n35 = Bundle By Name(cluster=T69 {"Autotune Gain"=refnum, "Target Amplitude [mV]"=refnum} ("Autotune Gain"), "Autotune Gain"=w405, "Target Amplitude [mV]"=w406) -> (w429:T69)
  n36 = Bundle By Name(cluster=T71 {"Pipette Offset"=refnum, "Offset Value [mV]"=refnum} ("Pipette Offset"), "Pipette Offset"=w416, "Offset Value [mV]"=w417) -> (w425:T71)
  n37 = Bundle By Name(cluster=T34 {"Current Signal"=refnum, "PSD"=refnum, "Pressure Signal"=refnum, "Current [nA]"=refnum, "Resistance [MOhm]"=refnum} ("Indicators"), "Resistance [MOhm]"=w41, "Current [nA]"=w42, "Current Signal"=w93, "PSD"=w46, "Pressure Signal"=w92) -> (w43:T34)
  n38 = Unbundle By Name(w88) -> ("Signals Sampling"=w87:T72, "Pressure Signal"=w86:T73, "Electrode Signals"=w45:T74)
  n39 = Bundle By Name(cluster=T70 {"Test Signal"=refnum, "Amplitude [mV]"=refnum, "Frequency [hz]"=refnum} ("Test Signal"), "Test Signal"=w413, "Amplitude [mV]"=w415, "Frequency [hz]"=w414) -> (w427:T70)
  n40 = call "Amplifier Daemon.vi"("Multiclamp Reference"=w89, "Signal"=w411, "Gain"=w412, "Autotune Gain"=w429, "Test Signal"=w427, "Error In"=w90, "Capacitance Compensation"=w431, "Pipette Offset"=w425, "Holding Potential"=w403, "Reset"=w400, "Exit"=w423) -> ("Error Out"=w106:errorcluster)  [unwired: 8 in]
  n41 = call "Signal Acquisition.vi"("Signals Sampling"=w87, "Pressure Signal"=w86, "Electrode Signals"=w45, "Indicators"=w43, "Filter"=w94, "Filter Led Indicator"=w95, "IIR filter specifications"=w96, "Exit"=w97) -> ("error out"=w85:errorcluster)  [unwired: 11 in]
  n42 = Merge Errors(w106, w85) -> (w107:errorcluster)
  n43 = control-ref of="Analyzer"() -> (w399:refnum<vi>)
  n44 = control-ref of="Auto Button"() -> (w326:refnum<vi>)
  n45 = control-ref of="Auto Led"() -> (w327:refnum<vi>)
  n46 = control-ref of="Load Pipette"() -> (w381:refnum<vi>)
  n47 = control-ref of="Drive In"() -> (w380:refnum<vi>)
  n48 = control-ref of="Hunt"() -> (w379:refnum<vi>)
  n49 = control-ref of="Seal"() -> (w382:refnum<vi>)
  n50 = control-ref of="Break In"() -> (w378:refnum<vi>)
  n51 = control-ref of="Abort"() -> (w40:refnum<vi>)
  n52 = control-ref of="Exit"() -> (w377:refnum<vi>)
  n53 = control-ref of="Holding Potential"() -> (w342:refnum<vi>)
  n54 = control-ref of="Reset"() -> (w331:refnum<vi>)
  n55 = control-ref of="Indicator"() -> (w362:refnum<vi>)
  n56 = control-ref of="Capacitance Compensation"() -> (w349:refnum<vi>)
  n57 = control-ref of="Disengage Tip"() -> (w361:refnum<vi>)
  n58 = control-ref of="Autotune Gain"() -> (w346:refnum<vi>)
  n59 = control-ref of="Activate Pressure"() -> (w390:refnum<vi>)
  n60 = control-ref of="Pulse"() -> (w389:refnum<vi>)
  n61 = control-ref of="Status"() -> (w398:refnum<vi>)
  n62 = control-ref of="Approach Indicator"() -> (w396:refnum<vi>)
  n63 = control-ref of="Zero"() -> (w395:refnum<vi>)
  n64 = control-ref of="Step"() -> (w394:refnum<vi>)
  n65 = control-ref of="Drive to"() -> (w393:refnum<vi>)
  n66 = control-ref of="Go to"() -> (w391:refnum<vi>)
  n67 = control-ref of="Pipette Offset"() -> (w367:refnum<vi>)
  n68 = control-ref of="Test Signal"() -> (w366:refnum<vi>)
  n69 = control-ref of="Test Signal"() -> (w350:refnum<vi>)
  n70 = control-ref of="Pressure SPs [KPa]"() -> (w336:refnum<vi>)
  n71 = control-ref of="Manipulator Dynamics"() -> (w363:refnum<vi>)
  n72 = control-ref of="Seal Parameters"() -> (w338:refnum<vi>)
  n73 = control-ref of="Suction Parameters"() -> (w340:refnum<vi>)
  n74 = control-ref of="Holding Potential Dynamics"() -> (w339:refnum<vi>)
  n75 = control-ref of="Current Position"() -> (w397:refnum<vi>)
  n76 = control-ref of="Resistance [MOhm]"() -> (w323:refnum<vi>)
  n77 = control-ref of="Current [nA]"() -> (w324:refnum<vi>)
  n78 = control-ref of="Blockage Threshold [%]"() -> (w371:refnum<vi>)
  n79 = control-ref of="Max Attempt"() -> (w372:refnum<vi>)
  n80 = control-ref of="R0/R2"() -> (w354:refnum<vi>)
  n81 = control-ref of="R1/R2"() -> (w353:refnum<vi>)
  n82 = control-ref of="R0/R1"() -> (w352:refnum<vi>)
  n83 = control-ref of="Target Amplitude [V]"() -> (w345:refnum<vi>)
  n84 = control-ref of="Length [ms]"() -> (w388:refnum<vi>)
  n85 = control-ref of="Voltage [mV]"() -> (w386:refnum<vi>)
  n86 = control-ref of="Pressure [KPa]"() -> (w384:refnum<vi>)
  n87 = control-ref of="Depth [um]"() -> (w392:refnum<vi>)
  n88 = control-ref of="Offset [mV]"() -> (w368:refnum<vi>)
  n89 = control-ref of="Amplitude [mV]"() -> (w365:refnum<vi>)
  n90 = control-ref of="Direction"() -> (w25:refnum<vi>)
  n91 = control-ref of="State"() -> (w330:refnum<vi>)
  n92 = control-ref of="Manipulator transformation"() -> (w337:refnum<vi>)
  n93 = control-ref of="Frequency [hz]"() -> (w364:refnum<vi>)
  n94 = control-ref of="Holding Potential [mV]"() -> (w341:refnum<vi>)
  n95 = control-ref of="Break in Thr [MOhm]"() -> (w325:refnum<vi>)
  n96 = control-ref of="Detection Thr [%]"() -> (w360:refnum<vi>)
  n97 = control-ref of="R0"() -> (w356:refnum<vi>)
  n98 = control-ref of="R1"() -> (w355:refnum<vi>)
  n99 = control-ref of="R2"() -> (w351:refnum<vi>)
  n100 = control-ref of="R0-R2"() -> (w357:refnum<vi>)
  n101 = control-ref of="Pressure Sp Manual [KPa]"() -> (w385:refnum<vi>)
  n102 = Bundle By Name(cluster=T66 {"On/Off"=refnum, "Pulse Controls"={"Pulse"=refnum, "Length [ms]"=refnum, "Voltage [mV]"=refnum, "Pulse Pressure [KPa]"=refnum}, "Pressure Sp Manual [KPa]"=refnum} ("Pressure Controls"), "On/Off"=w390, "Pressure Sp Manual [KPa]"=w385, "Pulse Controls.Pulse"=w389, "Pulse Controls.Length [ms]"=w388, "Pulse Controls.Voltage [mV]"=w386, "Pulse Controls.Pulse Pressure [KPa]"=w384) -> (w383:T66)
  n103 = Bundle By Name(cluster=T58 {"Suction Parameters"=refnum, "Holding Potential Dynamics"=refnum, "Seal Parameters"=refnum} ("Seal Dynamics"), "Seal Parameters"=w338, "Suction Parameters"=w340, "Holding Potential Dynamics"=w339) -> (w332:T58)
  n104 = Bundle By Name(cluster=T59 {"Test Signal Levels"=refnum, "Pressure Levels [KPa]"=refnum} ("Calibration levels"), "Test Signal Levels"=w350, "Pressure Levels [KPa]"=w336) -> (w334:T59)
  n105 = Bundle By Name(cluster=T61 {"Autotune Gain"=refnum, "Target Amplitude [V]"=refnum} ("Autotune Gain"), "Autotune Gain"=w346, "Target Amplitude [V]"=w345) -> (w347:T61)
  n106 = Bundle By Name(cluster=T65 {"On/Off"=refnum, "Resistance [MOhm]"=refnum, "Current [pA]"=refnum} ("Signals"), "On/Off"=w399, "Resistance [MOhm]"=w323, "Current [pA]"=w324) -> (w375:T65)
  n107 = Bundle By Name(cluster=T64 {"Blockage Threshold"=refnum, "Max Attempt"=refnum} ("Unblockage Parameters"), "Blockage Threshold"=w371, "Max Attempt"=w372) -> (w373:T64)
  n108 = Bundle By Name(cluster=T31 {"Status"=refnum, "Position"=refnum, "Zero"=refnum, "Step"=refnum, "Localize"=refnum, "Approach Indicator"=refnum, "Depth [um]"=refnum, "Drive to Zero"=refnum, "Direction"=refnum} ("Manipulator Controllers"), "Status"=w398, "Position"=w397, "Approach Indicator"=w396, "Zero"=w395, "Step"=w394, "Localize"=w393, "Depth [um]"=w392, "Drive to Zero"=w391, "Direction"=w25) -> (w24:T31)
  n109 = Bundle By Name(cluster=T63 {"Pipette Offset"=refnum, "Offset"=refnum, "Test Signal"=refnum, "Amplitude [mV]"=refnum, "Frequency [hz]"=refnum} ("Test Signal Parameters and Offset"), "Pipette Offset"=w367, "Offset"=w368, "Test Signal"=w366, "Amplitude [mV]"=w365, "Frequency [hz]"=w364) -> (w369:T63)
  n110 = Bundle By Name(cluster=T60 {"ON/OFF"=refnum, "Controller [mV]"=refnum} ("Holding Potential Controls"), "ON/OFF"=w342, "Controller [mV]"=w341) -> (w343:T60)
  n111 = Bundle By Name(cluster=T30 {"Load Pipette"=refnum, "Drive In"=refnum, "Hunt"=refnum, "Seal"=refnum, "Break In"=refnum, "Abort"=refnum, "Exit"=refnum, "Auto"=refnum, "Auto Button"=refnum} ("Controls"), "Auto Button"=w326, "Auto"=w327, "Load Pipette"=w381, "Drive In"=w380, "Hunt"=w379, "Seal"=w382, "Break In"=w378, "Abort"=w40, "Exit"=w377) -> (w328:T30)
  n112 = Bundle By Name(cluster=T62 {"R(Z=0)"=refnum, "R(Z=-1)"=refnum, "R(Z=-2)"=refnum, "R0-R2"=refnum, "R0/R2 [%]"=refnum, "R1/R2 [%]"=refnum, "R0/R1 [%]"=refnum} ("Sensed Resistance Levels"), "R(Z=0)"=w356, "R(Z=-1)"=w355, "R(Z=-2)"=w351, "R0-R2"=w357, "R0/R2 [%]"=w354, "R1/R2 [%]"=w353, "R0/R1 [%]"=w352) -> (w358:T62)
  n113 = call "Autopatcher Daemon.vi"("Controls"=w328, "Break in Thr [MOhm]"=w325, "Detection Thr [%]"=w360, "Disengage Target"=w361, "Manipulator Dynamics"=w363, "Unblockage Parameters"=w373, "Sensed Resistance Levels"=w358, "Signals"=w375, "Pressure Controls"=w383, "Holding Potential Controls"=w343, "Autotune Gain"=w347, "Calibration levels"=w334, "Manipulator Controllers"=w24, "Capacitance Compensation"=w349, "Test and Offset Controls"=w369, "Dialog Indicator"=w362, "Seal Dynamics"=w332, "Reset"=w331, "Manipulator Transformation Matrix"=w337, "State"=w330) -> ("Error Out"=w174:errorcluster)  [unwired: 7 in]
  n114 = Merge Errors(w174, w107) -> (w175:errorcluster)
  n115 = control-ref of="Image"() -> (w179:refnum<vi>)
  n116 = control-ref of="Time Stamp"() -> (w142:refnum<vi>)
  n117 = control-ref of="Auto Button"() -> (w22:refnum<vi>)
  n118 = control-ref of="Auto Led"() -> (w21:refnum<vi>)
  n119 = control-ref of="Load Pipette"() -> (w15:refnum<vi>)
  n120 = control-ref of="Drive In"() -> (w16:refnum<vi>)
  n121 = control-ref of="Hunt"() -> (w17:refnum<vi>)
  n122 = control-ref of="Seal"() -> (w14:refnum<vi>)
  n123 = control-ref of="Break In"() -> (w18:refnum<vi>)
  n124 = control-ref of="Abort"() -> (w23:refnum<vi>)
  n125 = control-ref of="Exit"() -> (w19:refnum<vi>)
  n126 = control-ref of="Scope Zero"() -> (w177:refnum<vi>)
  n127 = control-ref of="Drive to Position"() -> (w78:refnum<vi>)
  n128 = control-ref of="Calibrate FOV"() -> (w187:refnum<vi>)
  n129 = control-ref of="Calibrate Azimut"() -> (w70:refnum<vi>)
  n130 = control-ref of="Calibrate Elevation"() -> (w186:refnum<vi>)
  n131 = control-ref of="Autocalibration"() -> (w185:refnum<vi>)
  n132 = control-ref of="Acquire Initial Point"() -> (w184:refnum<vi>)
  n133 = control-ref of="Acquire Final Point"() -> (w183:refnum<vi>)
  n134 = control-ref of="Align Trajectory"() -> (w192:refnum<vi>)
  n135 = control-ref of="Axial Approach"() -> (w191:refnum<vi>)
  n136 = control-ref of="Engage Target"() -> (w64:refnum<vi>)
  n137 = control-ref of="Indicator"() -> (w68:refnum<vi>)
  n138 = control-ref of="Abort"() -> (w38:refnum<vi>)
  n139 = control-ref of="Exit"() -> (w190:refnum<vi>)
  n140 = control-ref of="Status"() -> (w200:refnum<vi>)
  n141 = control-ref of="Approach Indicator"() -> (w199:refnum<vi>)
  n142 = control-ref of="Zero"() -> (w198:refnum<vi>)
  n143 = control-ref of="Step"() -> (w195:refnum<vi>)
  n144 = control-ref of="Drive to"() -> (w197:refnum<vi>)
  n145 = control-ref of="Go to"() -> (w196:refnum<vi>)
  n146 = control-ref of="Axial Approach"() -> (w203:refnum<vi>)
  n147 = control-ref of="Acquire Tip"() -> (w207:refnum<vi>)
  n148 = control-ref of="Disengage Tip"() -> (w206:refnum<vi>)
  n149 = control-ref of="Tip Indicator"() -> (w208:refnum<vi>)
  n150 = control-ref of="Focus Tip"() -> (w71:refnum<vi>)
  n151 = control-ref of="Acquire Target"() -> (w160:refnum<vi>)
  n152 = control-ref of="Disengage Target"() -> (w205:refnum<vi>)
  n153 = control-ref of="Target Indicator"() -> (w210:refnum<vi>)
  n154 = control-ref of="Focus Target"() -> (w72:refnum<vi>)
  n155 = control-ref of="Status"() -> (w145:refnum<vi>)
  n156 = control-ref of="Target Update"() -> (w144:refnum<vi>)
  n157 = control-ref of="Focus Button"() -> (w141:refnum<vi>)
  n158 = control-ref of="Start Coordinates [pix]"() -> (w1:refnum<vi>)
  n159 = control-ref of="Scope Current Position"() -> (w180:refnum<vi>)
  n160 = control-ref of="Scope Destination"() -> (w176:refnum<vi>)
  n161 = control-ref of="FOV indicator"() -> (w189:refnum<vi>)
  n162 = control-ref of="Angles"() -> (w188:refnum<vi>)
  n163 = control-ref of="Coorection Factor"() -> (w136:refnum<vi>)
  n164 = control-ref of="Current Position"() -> (w202:refnum<vi>)
  n165 = control-ref of="Destination Position"() -> (w201:refnum<vi>)
  n166 = control-ref of="Manipulator Dynamics"() -> (w194:refnum<vi>)
  n167 = control-ref of="Tip Coordinates"() -> (w209:refnum<vi>)
  n168 = control-ref of="Target Coordinates"() -> (w211:refnum<vi>)
  n169 = control-ref of="Traced Object [um]"() -> (w146:refnum<vi>)
  n170 = control-ref of="Start Coordinates [pix]"() -> (w137:refnum<vi>)
  n171 = control-ref of="Target\nDistance [um]"() -> (w66:refnum<vi>)
  n172 = control-ref of="Approach Factor [um]"() -> (w172:refnum<vi>)
  n173 = control-ref of="Final Clearance [um]"() -> (w171:refnum<vi>)
  n174 = control-ref of="Stability Delay [ms]"() -> (w170:refnum<vi>)
  n175 = control-ref of="Axial distance to cover [um]"() -> (w67:refnum<vi>)
  n176 = control-ref of="Depth [um]"() -> (w204:refnum<vi>)
  n177 = control-ref of="Timeout [ms]"() -> (w139:refnum<vi>)
  n178 = control-ref of="Max Attempts"() -> (w138:refnum<vi>)
  n179 = control-ref of="Area"() -> (w77:refnum<vi>)
  n180 = control-ref of="Cntr"() -> (w53:refnum<vi>)
  n181 = control-ref of="Direction"() -> (w9:refnum<vi>)
  n182 = control-ref of="Method"() -> (w140:refnum<vi>)
  n183 = control-ref of="State"() -> (w27:refnum<vi>)
  n184 = control-ref of="Scope Transformation Matrix"() -> (w178:refnum<vi>)
  n185 = control-ref of="Manipulator transformation"() -> (w193:refnum<vi>)
  n186 = control-ref of="All Objects [pix]"() -> (w59:refnum<vi>)
  n187 = control-ref of="Zoom"() -> (w48:refnum<vi>)
  n188 = control-ref of="Target Update Method"() -> (w143:refnum<vi>)
  n189 = Bundle By Name(cluster=T36 {"Focused Plane"={"Focus"=refnum, "Timeout"=refnum, "Max Attempts"=refnum, "Method"=refnum}, "Time Stamp"=refnum, "Visual Target"={"Coordinates [um]"=refnum, "Status"=refnum, "Update"=refnum, "Update Method"=refnum, "Start Coordinates [pix]"=refnum, "Area"=refnum, "Contrast"=refnum}, "Visible Objects [pix]"=refnum} ("Focus and Tracking"), "Visual Target.Coordinates [um]"=w146, "Visual Target.Status"=w145, "Visual Target.Update"=w144, "Visual Target.Update Method"=w143, "Time Stamp"=w142, "Focused Plane.Focus"=w141, "Focused Plane.Method"=w140, "Focused Plane.Timeout"=w139, "Focused Plane.Max Attempts"=w138, "Visible Objects [pix]"=w59, "Visual Target.Start Coordinates [pix]"=w137, "Visual Target.Area"=w77, "Visual Target.Contrast"=w53) -> (w54:T36)
  n190 = Bundle By Name(cluster=T39 {"Exit"=refnum, "Abort"=refnum, "Align Trajectory"=refnum, "Axial Approach"=refnum, "Dialog Indicator"=refnum, "Approach Target"=refnum, "Target\nDistance [um]"=refnum, "Axial distance\nto cover [um]"=refnum} ("Main Interface"), "Target\nDistance [um]"=w66, "Axial distance\nto cover [um]"=w67, "Align Trajectory"=w192, "Axial Approach"=w191, "Approach Target"=w64, "Dialog Indicator"=w68, "Abort"=w38, "Exit"=w190) -> (w65:T39)
  n191 = Bundle By Name(cluster=T29 {"Indicators"={"Current Pos"=refnum, "Destination"=refnum, "Status"=refnum, "Axial Approach"=refnum}, "Settings"={"Dynamics"=refnum, "Transformation"=refnum, "Direction"=refnum}, "Controls"={"Zero"=refnum, "Step"=refnum, "Drive To"=refnum, "Go To"=refnum, "Axial"=refnum, "Depth [um]"=refnum}} ("Manipulator Interface"), "Indicators.Current Pos"=w202, "Indicators.Destination"=w201, "Indicators.Status"=w200, "Indicators.Axial Approach"=w199, "Settings.Dynamics"=w194, "Settings.Transformation"=w193, "Controls.Zero"=w198, "Controls.Step"=w195, "Controls.Drive To"=w197, "Controls.Go To"=w196, "Controls.Axial"=w203, "Controls.Depth [um]"=w204, "Settings.Direction"=w9) -> (w10:T29)
  n192 = Bundle By Name(cluster=T47 {"Indicators"={"FOV"=refnum, "Angles"=refnum}, "Buttons"={"Cal FOV"=refnum, "Cal Azimut"=refnum, "Cal Elevation"=refnum, "Auto Cal"=refnum, "Acq Initial"=refnum, "Acq Final"=refnum}, "Stability Delay [ms]"=refnum, "Scale Coorection Factor"=refnum} ("Calibration"), "Indicators.FOV"=w189, "Indicators.Angles"=w188, "Buttons.Cal FOV"=w187, "Buttons.Cal Azimut"=w70, "Buttons.Cal Elevation"=w186, "Buttons.Auto Cal"=w185, "Buttons.Acq Initial"=w184, "Buttons.Acq Final"=w183, "Stability Delay [ms]"=w170, "Scale Coorection Factor"=w136) -> (w134:T47)
  n193 = Bundle By Name(cluster=T35 {"Current Pos"=refnum, "Image interface"=refnum, "Transformation Matrix"=refnum, "Zero"=refnum, "Destination"=refnum, "Drive to Position"=refnum, "Zoom"=refnum} ("System of Reference Interface"), "Current Pos"=w180, "Image interface"=w179, "Transformation Matrix"=w178, "Zero"=w177, "Destination"=w176, "Drive to Position"=w78, "Zoom"=w48) -> (w49:T35)
  n194 = Bundle By Name(cluster=T50 {"Approach  Factor"=refnum, "Final Clearance"=refnum} ("Guided Approach Calibration"), "Approach  Factor"=w172, "Final Clearance"=w171) -> (w182:T50)
  n195 = Bundle By Name(cluster=T40 {"Coordinates"=refnum, "Acquire"=refnum, "Disengage"=refnum, "Indicator"=refnum, "Focus Target"=refnum} ("Target"), "Coordinates"=w211, "Acquire"=w160, "Disengage"=w205, "Indicator"=w210, "Focus Target"=w72) -> (w73:T40)
  n196 = Bundle By Name(cluster=T30 {"Load Pipette"=refnum, "Drive In"=refnum, "Hunt"=refnum, "Seal"=refnum, "Break In"=refnum, "Abort"=refnum, "Exit"=refnum, "Auto"=refnum, "Auto Button"=refnum} ("Controls"), "Auto Button"=w22, "Auto"=w21, "Load Pipette"=w15, "Drive In"=w16, "Hunt"=w17, "Seal"=w14, "Break In"=w18, "Abort"=w23, "Exit"=w19) -> (w13:T30)
  n197 = Bundle By Name(cluster=T41 {"Coordinates"=refnum, "Acquire"=refnum, "Disengage"=refnum, "Indicator"=refnum, "Focus Tip"=refnum} ("Tip"), "Coordinates"=w209, "Acquire"=w207, "Disengage"=w206, "Indicator"=w208, "Focus Tip"=w71) -> (w75:T41)
  n198 = call "Targeting Unit.vi"("Main Interface"=w65, "Focus and Tracking"=w54, "Guided Approach"=w182, "Controls"=w13, "Start Coordinates [pix]"=w1, "Manipulator Interface"=w10, "Target"=w73, "Tip"=w75, "System of Reference Interface"=w49, "Calibration"=w134, "State"=w27) -> ("Error Out"=w212:errorcluster)  [unwired: 4 in]
  n199 = Merge Errors(w212, w175) -> (w434:errorcluster)
  n200 = local read "Hardware Configuration"() -> (w432:T26)
  n201 = local read "Hardware Configuration"() -> (w173:T26)
  n202 = control-ref of="Image"() -> (w282:refnum<vi>)
  n203 = control-ref of="Time Stamp"() -> (w164:refnum<vi>)
  n204 = control-ref of="Time Stamp"() -> (w213:refnum<vi>)
  n205 = control-ref of="Status"() -> (w216:refnum<vi>)
  n206 = control-ref of="Approach Indicator"() -> (w217:refnum<vi>)
  n207 = control-ref of="Zero"() -> (w229:refnum<vi>)
  n208 = control-ref of="Step"() -> (w228:refnum<vi>)
  n209 = control-ref of="Drive to"() -> (w227:refnum<vi>)
  n210 = control-ref of="Go to"() -> (w225:refnum<vi>)
  n211 = control-ref of="Axial Approach"() -> (w214:refnum<vi>)
  n212 = control-ref of="Abort"() -> (w39:refnum<vi>)
  n213 = control-ref of="Exit"() -> (w215:refnum<vi>)
  n214 = control-ref of="Pipette Crash"() -> (w267:refnum<vi>)
  n215 = control-ref of="Internal Calibration"() -> (w275:refnum<vi>)
  n216 = control-ref of="Load Calibration File"() -> (w276:refnum<vi>)
  n217 = control-ref of="Save current FOV"() -> (w274:refnum<vi>)
  n218 = control-ref of="Focus Button"() -> (w240:refnum<vi>)
  n219 = control-ref of="Focus Tip"() -> (w239:refnum<vi>)
  n220 = control-ref of="Focus Target"() -> (w241:refnum<vi>)
  n221 = control-ref of="Acquire Tip"() -> (w168:refnum<vi>)
  n222 = control-ref of="Drive to Zero"() -> (w238:refnum<vi>)
  n223 = control-ref of="Scope Zero"() -> (w237:refnum<vi>)
  n224 = control-ref of="Abort"() -> (w37:refnum<vi>)
  n225 = control-ref of="Exit"() -> (w236:refnum<vi>)
  n226 = control-ref of="Drive to Position"() -> (w169:refnum<vi>)
  n227 = control-ref of="Acquire Surface"() -> (w114:refnum<vi>)
  n228 = control-ref of="Find Shank"() -> (w266:refnum<vi>)
  n229 = control-ref of="Find Tip"() -> (w265:refnum<vi>)
  n230 = control-ref of="Auto Adjust Green"() -> (w256:refnum<vi>)
  n231 = control-ref of="Auto Adjust Red"() -> (w254:refnum<vi>)
  n232 = control-ref of="Auto Delay"() -> (w124:refnum<vi>)
  n233 = control-ref of="Image Analisys"() -> (w284:refnum<vi>)
  n234 = control-ref of="Object Tracking"() -> (w246:refnum<vi>)
  n235 = control-ref of="Status"() -> (w245:refnum<vi>)
  n236 = control-ref of="Indicator"() -> (w235:refnum<vi>)
  n237 = control-ref of="Current Position"() -> (w218:refnum<vi>)
  n238 = control-ref of="Manipulator Dynamics"() -> (w224:refnum<vi>)
  n239 = control-ref of="Destination Position"() -> (w47:refnum<vi>)
  n240 = control-ref of="Angles"() -> (w269:refnum<vi>)
  n241 = control-ref of="Scanning Direction"() -> (w262:refnum<vi>)
  n242 = control-ref of="Scan Area"() -> (w248:refnum<vi>)
  n243 = control-ref of="Optic Flow Options"() -> (w167:refnum<vi>)
  n244 = control-ref of="FOV indicator"() -> (w271:refnum<vi>)
  n245 = control-ref of="Tip Coordinates"() -> (w280:refnum<vi>)
  n246 = control-ref of="Target Coordinates"() -> (w281:refnum<vi>)
  n247 = control-ref of="Scope Current Position"() -> (w279:refnum<vi>)
  n248 = control-ref of="Scope Destination"() -> (w231:refnum<vi>)
  n249 = control-ref of="Traced Object [um]"() -> (w244:refnum<vi>)
  n250 = control-ref of="Start Coordinates [pix]"() -> (w243:refnum<vi>)
  n251 = control-ref of="Depth [um]"() -> (w226:refnum<vi>)
  n252 = control-ref of="Surface @"() -> (w117:refnum<vi>)
  n253 = control-ref of="Stability Delay [ms]"() -> (w263:refnum<vi>)
  n254 = control-ref of="Vertical Sections"() -> (w261:refnum<vi>)
  n255 = control-ref of="Fucusing step [um]"() -> (w264:refnum<vi>)
  n256 = control-ref of="Erosion Value"() -> (w249:refnum<vi>)
  n257 = control-ref of="Display-N"() -> (w260:refnum<vi>)
  n258 = control-ref of="Frames"() -> (w258:refnum<vi>)
  n259 = control-ref of="Objects detected"() -> (w283:refnum<vi>)
  n260 = control-ref of="Traced Objects"() -> (w272:refnum<vi>)
  n261 = control-ref of="Area"() -> (w79:refnum<vi>)
  n262 = control-ref of="Cntr"() -> (w56:refnum<vi>)
  n263 = control-ref of="Direction"() -> (w29:refnum<vi>)
  n264 = control-ref of="Manipulator transformation"() -> (w223:refnum<vi>)
  n265 = control-ref of="All Objects [pix]"() -> (w63:refnum<vi>)
  n266 = control-ref of="Traced Objects [pix]"() -> (w61:refnum<vi>)
  n267 = control-ref of="Transformation Matrix"() -> (w232:refnum<vi>)
  n268 = control-ref of="Objective"() -> (w268:refnum<vi>)
  n269 = control-ref of="Average"() -> (w259:refnum<vi>)
  n270 = control-ref of="Visualized Color Plane"() -> (w251:refnum<vi>)
  n271 = control-ref of="Zoom"() -> (w253:refnum<vi>)
  n272 = control-ref of="Delay"() -> (w252:refnum<vi>)
  n273 = control-ref of="Green Channel"() -> (w257:refnum<vi>)
  n274 = control-ref of="Red Channel"() -> (w255:refnum<vi>)
  n275 = control-ref of="Erosion Filter"() -> (w278:refnum<vi>)
  n276 = control-ref of="Analysis Plane"() -> (w273:refnum<vi>)
  n277 = Unbundle By Name(w173) -> ("Sciscan core Ref"=w161:path)
  n278 = Bundle By Name(cluster=T45 {"Display Every N"=refnum, "Average"=refnum, "Frames"=refnum, "Colour Plane"=refnum, "Zoom"=refnum, "Delay"=refnum, "Equalization"={"Green Channel"=refnum, "Auto Adjust Green"=refnum, "Red Channel"=refnum, "Auto Adjust Red"=refnum}, "Auto Delay"=refnum} ("Visualization Parameters"), "Display Every N"=w260, "Average"=w259, "Frames"=w258, "Colour Plane"=w251, "Zoom"=w253, "Delay"=w252, "Equalization.Green Channel"=w257, "Equalization.Auto Adjust Green"=w256, "Equalization.Red Channel"=w255, "Equalization.Auto Adjust Red"=w254, "Auto Delay"=w124) -> (w125:T45)
  n279 = Bundle By Name(cluster=T37 {"Object Tracking Command"=refnum, "Status Indicator"=refnum, "Start Coordinates [pix]"=refnum, "Traced Object [um]"=refnum, "Area"=refnum, "Contrast"=refnum} ("Unit"), "Traced Object [um]"=w244, "Object Tracking Command"=w246, "Status Indicator"=w245, "Start Coordinates [pix]"=w243, "Area"=w79, "Contrast"=w56) -> (w247:T37)
  n280 = Bundle By Name(cluster=T56 {"Internal Calibrated FOV"=refnum, "Load FOV calibration file"=refnum, "Save current FOV"=refnum} ("FOV controls"), "Internal Calibrated FOV"=w275, "Load FOV calibration file"=w276, "Save current FOV"=w274) -> (w162:T56)
  n281 = Bundle By Name(cluster=T53 {"Tip Coordinates"=refnum, "Target Coordinates"=refnum, "Scope Position"=refnum, "FOV"=refnum, "Scope Goto Position"=refnum} ("Indicators"), "FOV"=w271, "Tip Coordinates"=w280, "Target Coordinates"=w281, "Scope Position"=w279, "Scope Goto Position"=w231) -> (w233:T53)
  n282 = Bundle By Name(cluster=T38 {"On/Off"=refnum, "All Objects"=refnum, "Color Plane"=refnum, "Erosion"=refnum, "Traced Objects"=refnum, "Frame Time Stamp"=refnum, "Optic Flow Settings"=refnum, "All Object [pix]"=refnum, "Traced Object [pix]"=refnum} ("Image Analysis"), "On/Off"=w284, "Erosion"=w278, "All Objects"=w283, "Color Plane"=w273, "Traced Objects"=w272, "All Object [pix]"=w63, "Traced Object [pix]"=w61, "Frame Time Stamp"=w213, "Optic Flow Settings"=w167) -> (w60:T38)
  n283 = Bundle By Name(cluster=T54 {"Find Shank"=refnum, "Find Tip"=refnum, "Scanning Direction"=refnum, "Scan Area"=refnum, "Stability Delay [ms]"=refnum, "Vertical Steps"=refnum, "Fucusing step [um]"=refnum, "Erosion Value"=refnum} ("Exploration and Autofocus"), "Find Shank"=w266, "Find Tip"=w265, "Scanning Direction"=w262, "Scan Area"=w248, "Stability Delay [ms]"=w263, "Vertical Steps"=w261, "Fucusing step [um]"=w264, "Erosion Value"=w249) -> (w234:T54)
  n284 = Bundle By Name(cluster=T55 {"Angles"=refnum, "Objective Diameter"=refnum, "Pipette Crash"=refnum} ("Parameters for Legal Movements"), "Angles"=w269, "Objective Diameter"=w268, "Pipette Crash"=w267) -> (w163:T55)
  n285 = Unbundle By Name(w432) -> ("Manipulator Port"=w230:refnum<visa-resource-name>)
  n286 = Bundle By Name(cluster=T51 {"Approach"=refnum, "Status"=refnum, "Current Position"=refnum} ("Manipulator Indicator"), "Status"=w216, "Approach"=w217, "Current Position"=w218) -> (w219:T51)
  n287 = Bundle By Name(cluster=T43 {"Focus Tip"=refnum, "Focus Target"=refnum, "Drive to Zero"=refnum, "Zero"=refnum, "Acquire Tip"=refnum, "Focus Button"=refnum, "Exit"=refnum, "Abort"=refnum, "Drive to"=refnum, "Surface @"=refnum, "Acquire Surface"=refnum} ("Buttons"), "Focus Button"=w240, "Focus Tip"=w239, "Focus Target"=w241, "Acquire Tip"=w168, "Drive to Zero"=w238, "Zero"=w237, "Abort"=w37, "Exit"=w236, "Drive to"=w169, "Surface @"=w117, "Acquire Surface"=w114) -> (w115:T43)
  n288 = Bundle By Name(cluster=T52 {"Dynamics"=refnum, "Transformation"=refnum} ("Manipulator Settings"), "Transformation"=w223, "Dynamics"=w224) -> (w221:T52)
  n289 = To Variant(anything=w282) -> (Variant=w105:variant)
  n290 = Bundle By Name(cluster=T32 {"Zero"=refnum, "Step"=refnum, "Go to"=refnum, "Drive to Depth"=refnum, "Exit"=refnum, "Abort"=refnum, "Depth [um]"=refnum, "Dest Position"=refnum, "Axial"=refnum, "Direction"=refnum} ("Commands"), "Zero"=w229, "Step"=w228, "Drive to Depth"=w227, "Depth [um]"=w226, "Go to"=w225, "Dest Position"=w47, "Axial"=w214, "Abort"=w39, "Exit"=w215, "Direction"=w29) -> (w28:T32)
  n291 = control-ref of="Start Coordinates [pix] 2"() -> ()  [unwired: 1 out]
  n292 = call "IMAQ Create"("Image Name"="Vision Frame") -> ("New Image"=w109:T14, "error out"=w4:errorcluster)  [unwired: 4 in]
  n293 = call "IMAQ Create"("Image Name"="Input Frame") -> ("New Image"=w5:T14, "error out"=w6:errorcluster)  [unwired: 4 in]
  n294 = Build Array(w247) -> (w57:T75)
  n295 = call "Manipulator Daemon.vi"("Manipulator Indicator"=w219, "Manipulator Settings"=w221, "Commands"=w28, "VISA resource in"=w230) -> ("Error Out"=w12:errorcluster)  [unwired: 7 in]
  n296 = call "Scope Daemon.vi"("Sciscan core Ref"=w161, "Buttons"=w115, "Indicators"=w233, "Visualization Parameters"=w125, "Current Frame"=w5, "Frame Time Stamp"=w164, "error in (no error)"=w6, "Transformation Matrix"=w232, "FOV controls"=w162, "Parameters for Legal Movements"=w163) -> ("Current Frame Out"=w7:T14, "error out"=w8:errorcluster)  [unwired: 4 in]
  n297 = call "Visual Analyser.vi"("Image In (RGB overlay)"=w5, "Buttons"=w115, "Indicators"=w233, "Dialog Indicator"=w235, "Vision Frame"=w109, "Image Indicator"=w105, "Visualization Parameters"=w125, "Image Analysis"=w60, "Error In"=w4, "Exploration and Autofocus"=w234, "Targeting Units"=w57, "Transformation Matrix"=w232) -> ("Vision Frame Out"=w2:T14, "Error Out"=w3:errorcluster)  [unwired: 2 in]
  n298 = call "IMAQ Dispose"("Image"=w7, "error in (no error)"=w8) -> ("error out"=w165:errorcluster)  [unwired: 4 in]
  n299 = call "IMAQ Dispose"("Image"=w2, "error in (no error)"=w3) -> ("error out"=w104:errorcluster)  [unwired: 4 in]
  n300 = Merge Errors(w12, w165, w104, w434) -> (w322:errorcluster)
  n301 = local read "Hardware Configuration"() -> (w311:T26)
  n302 = local read "Hardware Configuration"() -> (w82:T26)
  n303 = Unbundle By Name(w311) -> ("Signals Sampling.Samples Number"=w310:i32, "Signals Sampling.Sampling frequecy [hz]"=w308:dbl)
  n304 = control-ref of="Resistance"() -> (w289:refnum<vi>)
  n305 = control-ref of="Current"() -> (w288:refnum<vi>)
  n306 = control-ref of="Holding Potential"() -> (w287:refnum<vi>)
  n307 = control-ref of="Pressure"() -> (w286:refnum<vi>)
  n308 = control-ref of="Position"() -> (w285:refnum<vi>)
  n309 = control-ref of="Test Signal"() -> (w313:refnum<vi>)
  n310 = control-ref of="Current"() -> (w294:refnum<vi>)
  n311 = control-ref of="Current"() -> (w321:refnum<vi>)
  n312 = control-ref of="Resistance"() -> (w320:refnum<vi>)
  n313 = control-ref of="Resistance"() -> (w297:refnum<vi>)
  n314 = control-ref of="Holding Potential Chart"() -> (w293:refnum<vi>)
  n315 = control-ref of="Pressure Signal"() -> (w91:refnum<vi>)
  n316 = control-ref of="Report Image"() -> (w128:refnum<vi>)
  n317 = control-ref of="Time Stamp"() -> (w127:refnum<vi>)
  n318 = control-ref of="Trajectory"() -> (w129:refnum<vi>)
  n319 = control-ref of="Exit"() -> (w319:refnum<vi>)
  n320 = control-ref of="Valves"() -> (w149:refnum<vi>)
  n321 = control-ref of="Positive Branch"() -> (w151:refnum<vi>)
  n322 = control-ref of="Negative Branch"() -> (w150:refnum<vi>)
  n323 = control-ref of="Activate Pressure"() -> (w148:refnum<vi>)
  n324 = control-ref of="Exit"() -> (w153:refnum<vi>)
  n325 = control-ref of="Pulse"() -> (w147:refnum<vi>)
  n326 = control-ref of="REC"() -> (w295:refnum<vi>)
  n327 = control-ref of="Record Button"() -> (w298:refnum<vi>)
  n328 = control-ref of="Exit"() -> (w299:refnum<vi>)
  n329 = control-ref of="Play Button"() -> (w123:refnum<vi>)
  n330 = control-ref of="Report Plot"() -> (w290:refnum<vi>)
  n331 = control-ref of="Vision Overlay"() -> (w108:refnum<vi>)
  n332 = control-ref of="Exit"() -> (w292:refnum<vi>)
  n333 = control-ref of="Analyzer"() -> (w302:refnum<vi>)
  n334 = control-ref of="Filter"() -> (w305:refnum<vi>)
  n335 = control-ref of="Exit"() -> (w304:refnum<vi>)
  n336 = control-ref of="Pressure Controller Dynamics"() -> (w83:refnum<vi>)
  n337 = control-ref of="Angles"() -> (w118:refnum<vi>)
  n338 = control-ref of="Calibration Parameters"() -> (w120:refnum<vi>)
  n339 = control-ref of="Geometrical Transformation"() -> (w119:refnum<vi>)
  n340 = control-ref of="Current Position"() -> (w111:refnum<vi>)
  n341 = control-ref of="Tip Coordinates"() -> (w33:refnum<vi>)
  n342 = control-ref of="Target Coordinates"() -> (w32:refnum<vi>)
  n343 = control-ref of="IIR Filter Specifications"() -> (w303:refnum<vi>)
  n344 = control-ref of="Resistance [MOhm]"() -> (w314:refnum<vi>)
  n345 = control-ref of="Current [nA]"() -> (w315:refnum<vi>)
  n346 = control-ref of="Length [ms]"() -> (w157:refnum<vi>)
  n347 = control-ref of="Voltage [mV]"() -> (w155:refnum<vi>)
  n348 = control-ref of="Pressure [KPa]"() -> (w156:refnum<vi>)
  n349 = control-ref of="Surface @"() -> (w34:refnum<vi>)
  n350 = control-ref of="Amplitude [mV]"() -> (w112:refnum<vi>)
  n351 = control-ref of="State"() -> (w36:refnum<vi>)
  n352 = control-ref of="Detection Thr [%]"() -> (w316:refnum<vi>)
  n353 = control-ref of="R0"() -> (w317:refnum<vi>)
  n354 = control-ref of="R2"() -> (w318:refnum<vi>)
  n355 = control-ref of="Pressure Sp Manual [KPa]"() -> (w98:refnum<vi>)
  n356 = control-ref of="File Path Control"() -> (w296:refnum<vi>)
  n357 = control-ref of="File Path Control"() -> (w291:refnum<vi>)
  n358 = control-ref of="Visualized Color Plane"() -> (w52:refnum<vi>)
  n359 = control-ref of="Slider"() -> (w132:refnum<vi>)
  n360 = control-ref of="Loading Bar"() -> (w51:refnum<vi>)
  n361 = control-ref of="Gain"() -> (w113:refnum<vi>)
  n362 = Bundle By Name(cluster=T49 {"Length [ms]"=refnum, "Pressure [KPa] Closed Loop"=refnum, "Voltage [mV] Open Loop"=refnum} ("Pulse Dynamics"), "Length [ms]"=w157, "Voltage [mV] Open Loop"=w155, "Pressure [KPa] Closed Loop"=w156) -> (w158:T49)
  n363 = Bundle By Name(cluster=T42 {"Pulse Dynamics"={"Length [ms]"=refnum, "Pressure [KPa] Closed Loop"=refnum, "Voltage [mV] Open Loop"=refnum}, "On/Off"=refnum, "Exit"=refnum, "Pulse"=refnum, "Pressure Sp [KPa]"=refnum, "Pressure Controller Dynamics"=refnum} ("Controls"), "Pressure Sp [KPa]"=w98, "On/Off"=w148, "Pressure Controller Dynamics"=w83, "Exit"=w153, "Pulse"=w147, "Pulse Dynamics"=w158) -> (w81:T42)
  n364 = Unbundle By Name(w82) -> ("Pressure Controller Port"=w80:refnum<visa-resource-name>)
  n365 = Bundle By Name(cluster=T33 {"Current"=refnum, "Holding Potential"=refnum, "Recording indicator"=refnum, "Pressure"=refnum, "Resistance"=refnum, "Manipulator Position"=refnum, "Tip Coordinates"=refnum, "Target Coordinates"=refnum, "Surface in Space [um]"=refnum, "State"=refnum} ("Indicators"), "Resistance"=w297, "Current"=w294, "Holding Potential"=w293, "Pressure"=w91, "Manipulator Position"=w111, "State"=w36, "Recording indicator"=w295, "Surface in Space [um]"=w34, "Tip Coordinates"=w33, "Target Coordinates"=w32) -> (w31:T33)
  n366 = Bundle By Name(cluster=T57 {"On/Off"=refnum, "Filter On/Off"=refnum, "Exit"=refnum, "IIR filter specifications"=refnum} ("Controllers"), "On/Off"=w302, "Filter On/Off"=w305, "Exit"=w304, "IIR filter specifications"=w303) -> (w306:T57)
  n367 = Bundle By Name(cluster=T46 {"Resistance"=refnum, "Current"=refnum, "Pressure"=refnum, "Holding Potential"=refnum, "Position"=refnum, "Trajectory"=refnum} ("Indicators"), "Resistance"=w289, "Current"=w288, "Holding Potential"=w287, "Pressure"=w286, "Position"=w285, "Trajectory"=w129) -> (w130:T46)
  n368 = Bundle By Name(cluster=T44 {"Angles"=refnum, "Calibration"=refnum, "Transformation"=refnum} ("Configuration"), "Angles"=w118, "Calibration"=w120, "Transformation"=w119) -> (w121:T44)
  n369 = Bundle By Name(cluster=T48 {"Valves"=refnum, "Branch +"=refnum, "Branch -"=refnum} ("Indicators"), "Valves"=w149, "Branch +"=w151, "Branch -"=w150) -> (w152:T48)
  n370 = Multiply(x=1000, y=w310) -> (x*y=w307:i32)
  n371 = Divide(x=w307, y=w308) -> (x/y=w300:dbl)
  n372 = To Variant(anything=w128) -> (Variant=w133:variant)
  n373 = call "Logger.vi"("Record"=w298, "Indicators"=w31, "Time Stamp"=w127, "Exit"=w299, "Visual Data"=w109, "File Path Control"=w296, "Configuration"=w121) -> ("error out"=w100:errorcluster)  [unwired: 8 in]
  n374 = To Quad Integer(1:w300) -> (0:w301:i64)
  n375 = call "Report Plotter.vi"("Plot"=w290, "Path"=w291, "Vision Overlay"=w108, "Indicators"=w130, "Play"=w123, "Exit"=w292, "Visualized Color Plane"=w52, "Slider"=w132, "Image Indicator"=w133, "Loading Bar"=w51) -> ("error out"=w101:errorcluster)  [unwired: 5 in]
  n376 = disable-structure shown="Disabled" {
    disable-tunnel: w313 -> [w442 _]
    disable-tunnel: w306 -> [w441 _]
    disable-tunnel: w301 -> [w440 _]
    disable-tunnel: _ -> [w439 _]
    disable-tunnel: _ -> [w438 _]
    disable-tunnel: w113 -> [w437 _]
    disable-tunnel: w112 -> [w436 _]
    disable-tunnel: [w435 _] -> w102
    frame Disabled {
      n377 = call "Signal Analyzer.vi"("Period [ms]"=w440, "Current [pA]"=w439, "Controllers"=w441, "Resistance [MOhm]"=w438, "Amplitude [mV]"=w436, "Gain"=w437, "Test Signal"=w442) -> ("error out"=w435:errorcluster)  [unwired: 4 in]
    }
    frame Enabled {
    }
  }
  n378 = call "RI plotter.vi"("Resistance val"=w314, "Resistance Indicator"=w320, "Current Indicator"=w321, "Current val"=w315, "Detection Thr [%]"=w316, "R0"=w317, "R2"=w318, "Exit"=w319) -> ("error out"=w103:errorcluster)  [unwired: 7 in]
  n379 = call "Pressure Regulator.vi"("Indicators"=w152, "Pressure Controller Port"=w80, "Controls"=w81) -> ("error out"=w99:errorcluster)  [unwired: 8 in]
  n380 = Merge Errors(w99, w100, w101, w102, w103, w322) -> (w433:errorcluster)
  n381 = flat-sequence {
    tunnel: w433 -> [w443]
    frame #0 {
      n382 = local read "High Level Controls"() -> (w446:T10)
      n383 = Bundle By Name(cluster=w446, "Exit"=FALSE) -> (w445:T10)
      n384 = local write "High Level Controls"(w445) -> ()
      "Error Out" <- w443
    }
  }
